vi "主界面.vi"() -> ()   [LabVIEW 2010]
uses:
  全局量/试验配置信息.vi
  全局量/全局_配置.vi
  全局量/自动测试结果.vi
panel:
  out "配置文件路径 2":path
  out "配置文件目录 2":path
  in  "进度提示":string
  in  "加载配置文件列表":u16(ring)
  out "配置文件路径":path
  out "配置文件目录":path
  in  "通道及参数配置":bool
  in  "选项卡":enum32{"板卡类型I", "板卡类型II"}(tab)
  in  "单选_数字量输入":bool
  in  "单选_数字量输出":bool
  in  "单选_DSP输入":bool
  in  "单选_CAN检测":bool
  in  "单选_LAN检测":bool
  in  "单选_R232检测":bool
  in  "btn_数字输出":bool
  in  "btn_DSP输入":bool
  in  "btn_CAN总线":bool
  in  "btn_LAN总线":bool
  in  "btn_R232_485总线":bool
  in  "btn_开始检测":bool
  in  "btn_数字输入":bool
  in  "单选_R485检测":bool
  in  "单选_AD输入":bool
  out "数字量输入检测":bool
  out "数字量输出检测":bool
  out "模拟量DSP输入检测":bool
  out "模拟量AD输入检测":bool
  out "CAN总线检测":bool
  out "LAN总线检测":bool
  out "RS232总线检测":bool
  out "RS485总线检测":bool
  in  "btn_自动开始检测类型2":bool
  in  "函数类型 4":bool caption="y =f4(A1sin(2*π*A2)x+A3)"
  in  "函数类型 3":bool caption="y =f3(x)"
  in  "函数类型 2":bool caption="y =f2(x,A1,A2,t)"
  in  "函数类型 1":bool caption="y =f1(A1*x+A2)"
  out "函数类型4检测":bool
  out "函数类型3检测":bool
  out "函数类型2检测":bool
  out "函数类型1检测":bool
  in  "单选_函数类型4":bool
  in  "单选_函数类型3":bool
  in  "单选_函数类型2":bool
  in  "单选_函数类型1":bool
  in  "进度每次增加数":dbl
  in  "btn_二维码识别":bool
  out "退出？":bool
  in  "btn_退出":bool
  in  "btn_报告管理":bool
  in  "str_测试地点":string
  in  "str_测试人员":string
  in  "str_测试编号":string
  in  "str_报告编号":string
  # "板卡综合测试装置"
  # "板 卡 测 试 信 息"
  # "试验报告编号："
  # "测试板卡编号："
  # "板卡类型："
  # "测试人员："
  # "测试地点："
  # "自动测试"
  # "分步测试"
  # "测试\n项\n目"
  # "分步测试"
  # "自动测试"
  # "测试\n项\n目"
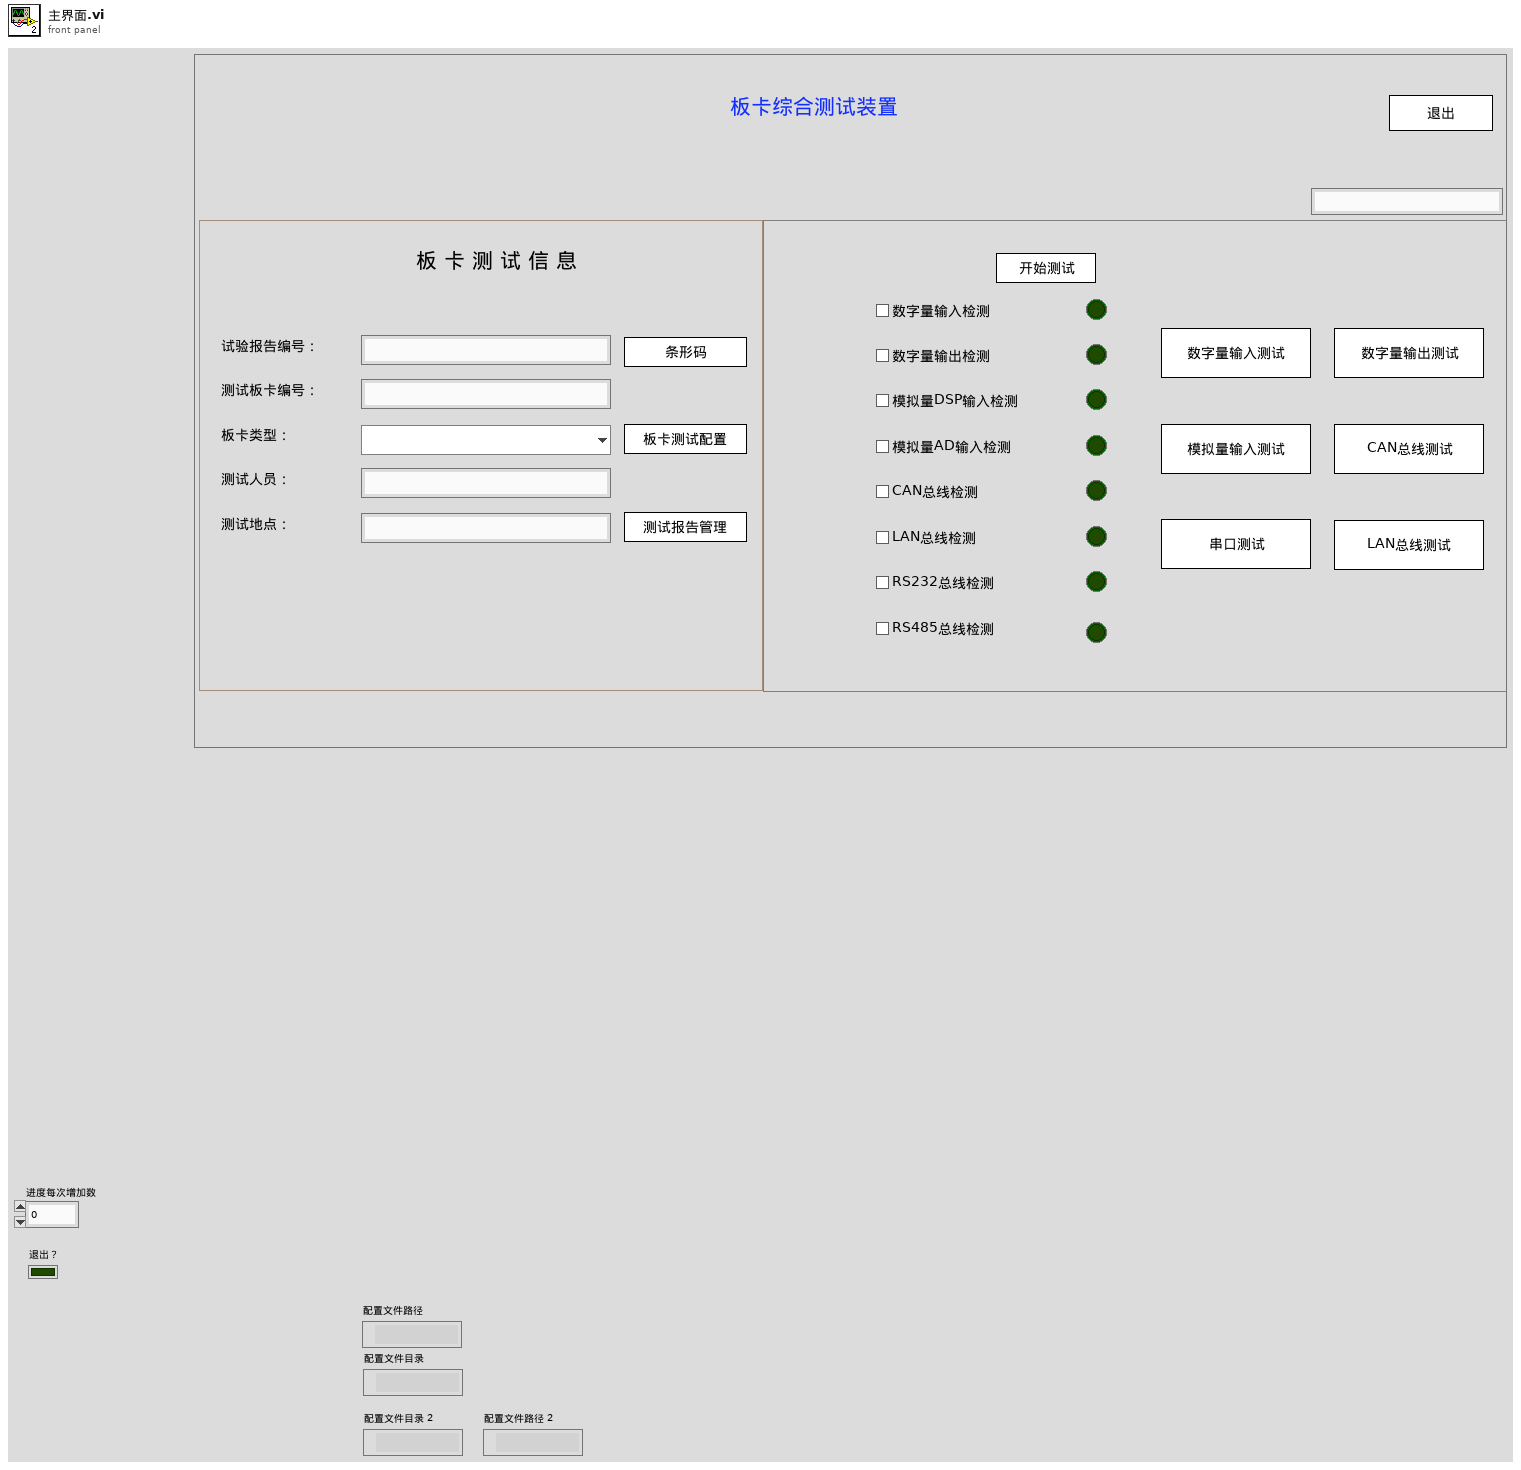
[diagram p1: front panel]
types:
  T1 = cluster{"数字量输入信号路数":i32, "数字量输出信号路数":i32, "DSP模拟量输入信号路数":u32, "DSP模拟量输入信号幅值":u32, "AD模拟量输入信号路数":u32, "AD模拟量输入信号幅值":u32, "RS232端口":u32, "RS232通信路数":u32, "RS232波特率":dbl, "RS485端口":u32, "RS485通信路数":u32, "RS485波特率":u32, "CAN通信路数":i32, "CAN波特率":u32, "以太网选择?":bool, "控制板IP":string, "以太网端口":u32}
  T2 = cluster{"str_报告编号":string, "str_测试编号":string, "RingText.Text":string, "str_测试人员":string, "str_测试地点":string}
  T3 = enum8{"Enabled", "Disabled", "Disabled and Grayed Out"}
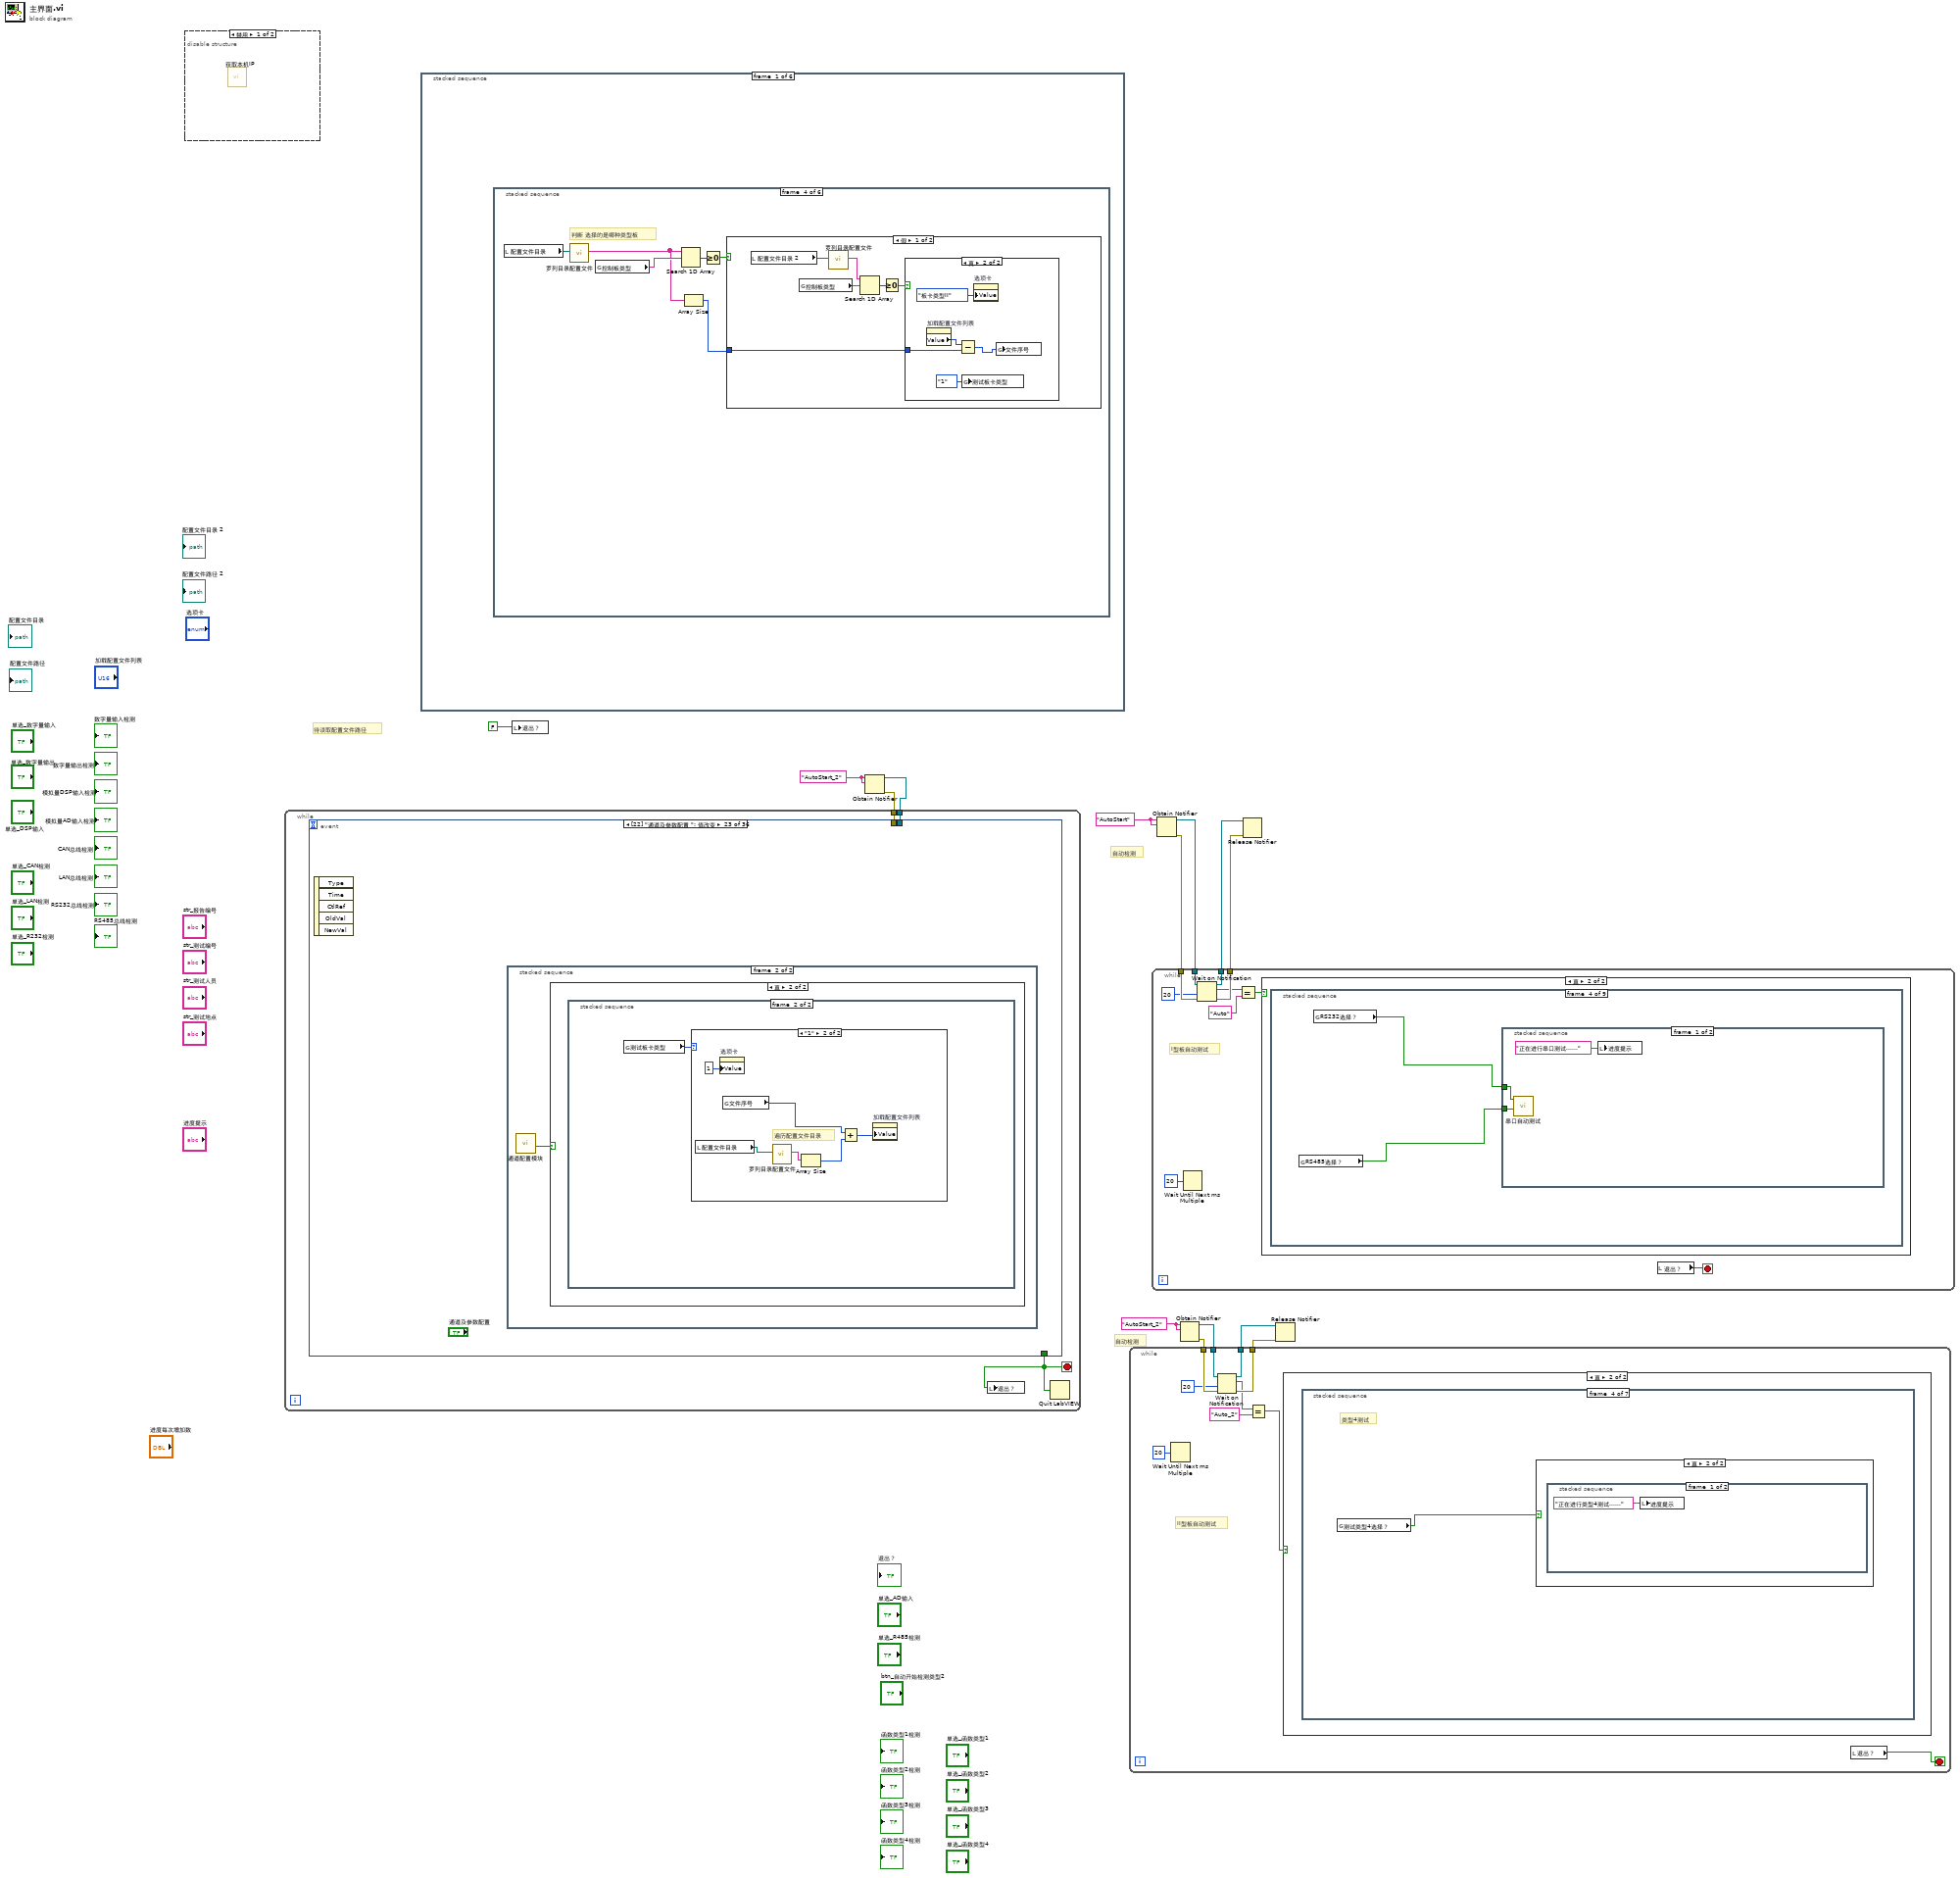
[diagram p0: block diagram]
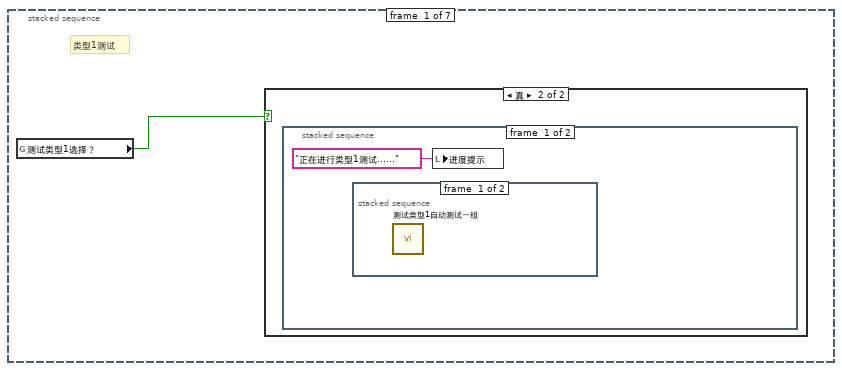
[diagram p4: hidden frame]
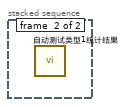
[diagram p6: hidden frame]
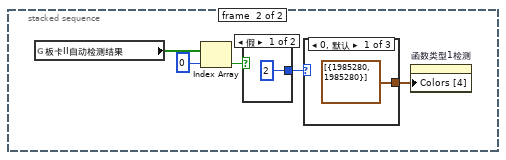
[diagram p7: hidden frame]
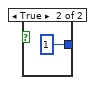
[diagram p8: hidden frame]
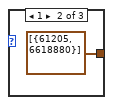
[diagram p9: hidden frame]
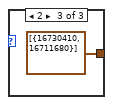
[diagram p10: hidden frame]
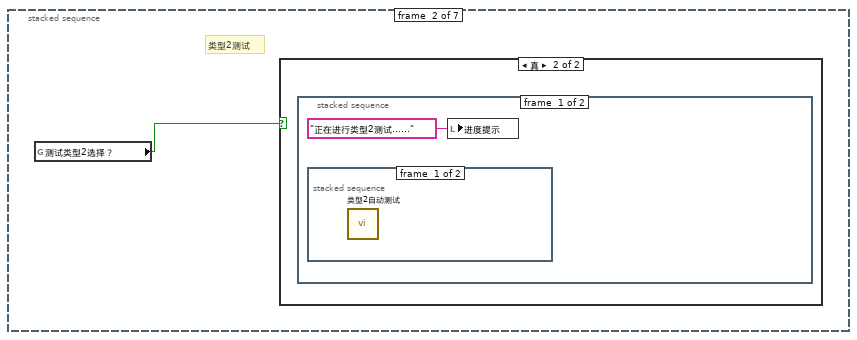
[diagram p11: hidden frame]
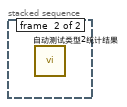
[diagram p13: hidden frame]
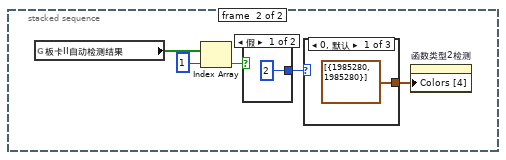
[diagram p14: hidden frame]
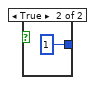
[diagram p15: hidden frame]
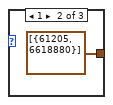
[diagram p16: hidden frame]
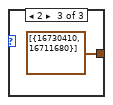
[diagram p17: hidden frame]
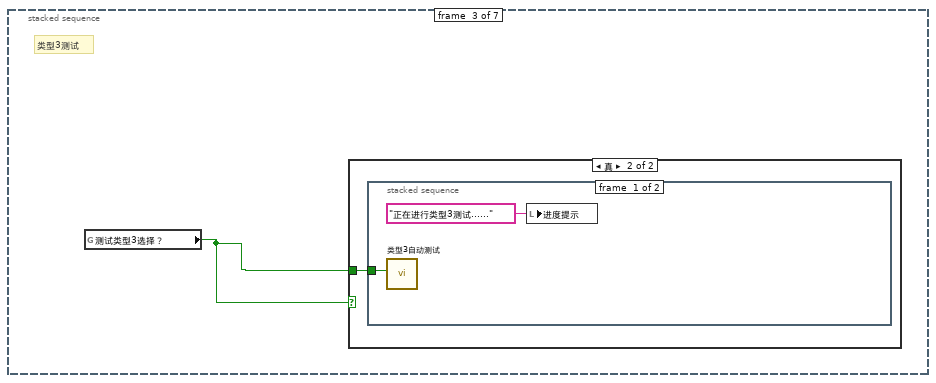
[diagram p18: hidden frame]
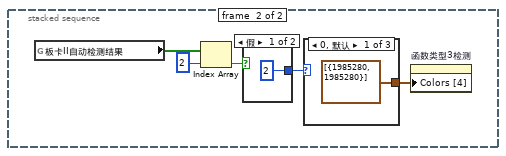
[diagram p20: hidden frame]
diagram:
  w4 = "AutoStart_2" ("名称（未命名）")
  w9 = "AutoStart_2" ("名称（未命名）")
  w14 = "AutoStart" ("名称（未命名）")
  # "待读取配置文件路径"
  # "自动检测"
  # "自动检测"
  n1 = disable-structure shown="禁用" {
    frame Disabled {
      n2 = call "获取本机IP.vi"() -> ()  [unwired: 9 in, 3 out]
    }
    frame Enabled {
    }
  }
  n3 = stacked-sequence {
    frame #0 {
      n4 = stacked-sequence {
        frame #0 {
          # "初始化配置文件路径"
          n5 = VI Library "VI库"() -> (path=w28:path)
          n6 = Strip Path(path=w28) -> (stripped path=w27:path)  [unwired: 1 out]
          n7 = Build Path(base path=w27, name or relative path="config" ("名称或相对路径")) -> (appended path=w16:path)
          n8 = Build Path(base path=w16, name or relative path="bordI_config" ("名称或相对路径")) -> (appended path=w22:path)
          n9 = Build Path(base path=w16, name or relative path="bordII_config" ("名称或相对路径")) -> (appended path=w19:path)
          n10 = call <vilib>:"Check if File or Folder Exists.vi"("path"=w22) -> ("file or folder exists?"=w23:bool, "dup path"=w24:path)  [unwired: 8 in, 1 out]
          n11 = call <vilib>:"Check if File or Folder Exists.vi"("path"=w19) -> ("file or folder exists?"=w18:bool, "dup path"=w17:path)  [unwired: 8 in, 1 out]
          n12 = case shown="假" w23 {
            tunnel: w24 -> [w32 w34]
            tunnel: [w33 w34] -> w21
            frame False {
              n13 = Create Folder(path (use dialog)=w32) -> (created path=w33:path)  [unwired: 2 in, 2 out]
            }
            frame True {
            }
          }
          n14 = case shown="假" w18 {
            tunnel: w17 -> [w29 w31]
            tunnel: [w30 w31] -> w20
            frame False {
              n15 = Create Folder(path (use dialog)=w29) -> (created path=w30:path)  [unwired: 2 in, 2 out]
            }
            frame True {
            }
          }
          n16 = local write "配置文件目录"(w21) -> ()
          n17 = local write "配置文件目录 2"(w20) -> ()
        }
        frame #1 {
          # "遍历配置文件目录"
          n18 = local read "配置文件目录"() -> (w39:path)
          n19 = local read "配置文件目录 2"() -> (w38:path)
          n20 = call "罗列目录配置文件.vi"("路径"=w39) -> ("数组"=w37:string[])  [unwired: 10 in]
          n21 = call "罗列目录配置文件.vi"("路径"=w38) -> ("数组"=w36:string[])  [unwired: 10 in]
          n22 = Insert Into Array(array=w37, new element=w36) -> (w35:string[])  [unwired: 1 in]
          n23 = property on="加载配置文件列表" class="Ring (严格)"("Strings []"=w35) -> ()  [unwired: 2 in, 2 out]
        }
        frame #2 {
          n24 = property on="加载配置文件列表" class="Ring (严格)"() -> ("RingText.Text"=w40:string)  [unwired: 2 in, 2 out]
          n25 = global write "试验配置信息.vi" "控制板类型"(w40) -> ()
        }
        frame #3 {
          # "判断 选择的是哪种类型板"
          n26 = local read "配置文件目录"() -> (w46:path)
          n27 = call "罗列目录配置文件.vi"("路径"=w46) -> ("数组"=w42:string[])  [unwired: 10 in]
          n28 = global read "试验配置信息.vi" "控制板类型"() -> (w45:string)
          n29 = Search 1D Array(1D array=w42, element=w45) -> (index of element=w44:i32)  [unwired: 1 in]
          n30 = Array Size(array=w42) -> (size(s)=w41:i32)
          n31 = Greater Or Equal To 0?(x=w44) -> (x >= 0?=w43:bool)
          n32 = case shown="假" w43 {
            tunnel: w41 -> [w47 _]
            frame False {
              n33 = local read "配置文件目录 2"() -> (w52:path)
              n34 = global read "试验配置信息.vi" "控制板类型"() -> (w51:string)
              n35 = call "罗列目录配置文件.vi"("路径"=w52) -> ("数组"=w50:string[])  [unwired: 10 in]
              n36 = Search 1D Array(1D array=w50, element=w51) -> (index of element=w49:i32)  [unwired: 1 in]
              n37 = Greater Or Equal To 0?(x=w49) -> (x >= 0?=w48:bool)
              n38 = case shown="真" w48 {
                tunnel: w47 -> [_ w54]
                frame False {
                }
                frame True {
                  n39 = property on="加载配置文件列表" class="Ring (严格)"() -> ("Value"=w56:u16)  [unwired: 2 in, 2 out]
                  n40 = Subtract(x=w56, y=w54) -> (x-y=w55:i32)
                  n41 = global write "试验配置信息.vi" "测试板卡类型"(enum16{"0", "1"}."1" ("测试板卡类型")) -> ()
                  n42 = property on="选项卡" class="TabCtl (严格)"("Value"=enum32{"板卡类型I", "板卡类型II"}."板卡类型II" ("选项卡")) -> ()  [unwired: 2 in, 2 out]
                  n43 = global write "试验配置信息.vi" "文件序号"(w55) -> ()
                }
              }
            }
            frame True {
              n44 = global write "试验配置信息.vi" "测试板卡类型"(enum16{"0", "1"}."0" ("测试板卡类型")) -> ()
              n45 = property on="选项卡" class="TabCtl (严格)"("Value"=enum32{"板卡类型I", "板卡类型II"}."板卡类型I" ("选项卡")) -> ()  [unwired: 2 in, 2 out]
              n46 = property on="加载配置文件列表" class="Ring (严格)"() -> ("Value"=w59:u16)  [unwired: 2 in, 2 out]
              n47 = global write "试验配置信息.vi" "文件序号"(w59) -> ()
            }
          }
        }
        frame #4 {
          # "待读取配置文件路径"
          n48 = local read "配置文件目录 2"() -> (w63:path)
          n49 = global read "试验配置信息.vi" "控制板类型"() -> (w61:string)
          n50 = Build Path(base path=w63, name or relative path=w61) -> (appended path=w62:path)
          n51 = local write "配置文件路径 2"(w62) -> ()
        }
        frame #5 {
          n52 = local read "配置文件路径 2"() -> (w66:path)
          n53 = call <vilib>:"Check if File or Folder Exists.vi"("path"=w66) -> ("file or folder exists?"=w65:bool, "dup path"=w64:path)  [unwired: 8 in, 1 out]
          n54 = case shown="真" w65 {
            tunnel: w64 -> [_ w67]
            frame False {
            }
            frame True {
              n55 = call "函数测试配置文件读取.vi"("配置文件路径"=w67) -> ("类型1路数"=w71:i32, "类型2路数"=w70:i32, "类型3路数"=w69:i32, "类型4路数"=w68:i32, "D_IN_1"=w75:string[][], "D_IN_2"=w74:string[][], "D_IN_3"=w73:string[][], "D_IN_4"=w72:string[][])  [unwired: 11 in]
              n56 = global write "试验配置信息.vi" "自测类型4路数"(w68) -> ()
              n57 = global write "试验配置信息.vi" "D_IN_1"(w75) -> ()
              n58 = global write "试验配置信息.vi" "D_IN_2"(w74) -> ()
              n59 = global write "试验配置信息.vi" "D_IN_3"(w73) -> ()
              n60 = global write "试验配置信息.vi" "D_IN_4"(w72) -> ()
              n61 = global write "试验配置信息.vi" "自测类型1路数"(w71) -> ()
              n62 = global write "试验配置信息.vi" "自测类型2路数"(w70) -> ()
              n63 = global write "试验配置信息.vi" "自测类型3路数"(w69) -> ()
            }
          }
        }
      }
    }
    frame #1 {
      n64 = global read "试验配置信息.vi" "控制板类型"() -> (w78:string)
      n65 = global write "全局_配置.vi" "CAN打开标志"(FALSE ("CAN打开标志")) -> ()
      n66 = local write "加载配置文件列表"(u16 0) -> ()
      n67 = call "读写配置文件.vi"("m_bCreat"=FALSE, "文件名称"=w78, "m_bRead"=TRUE) -> ("BoardConfig_output"=w92:T1)  [unwired: 8 in]
      n68 = Unbundle By Name(w92) -> ("数字量输入信号路数"=w86:i32, "数字量输出信号路数"=w85:i32, "DSP模拟量输入信号路数"=w84:u32, "DSP模拟量输入信号幅值"=w90:u32, "AD模拟量输入信号路数"=w83:u32, "AD模拟量输入信号幅值"=w87:u32, "RS232通信路数"=w82:u32, "RS232波特率"=w91:dbl, "RS485通信路数"=w81:u32, "CAN通信路数"=w80:i32)  [unwired: 7 out]
      n69 = global write "全局_配置.vi" "BoardConfig"(w92) -> ()
      n70 = global write "试验配置信息.vi" "测试板卡类型"(enum16{"0", "1"}."0" ("测试板卡类型")) -> ()
      n71 = case shown="0, 默认" w90 {
        tunnel: [3.3 10.0 24.0] -> w89
        frame 0, Default {
        }
        frame 1 {
        }
        frame 2 {
        }
      }
      n72 = case shown="2" w87 {
        tunnel: [6.0 10.0 24.0] -> w88
        frame 0, Default {
        }
        frame 1 {
        }
        frame 2 {
        }
      }
      n73 = global write "全局_配置.vi" "模拟量误差"(w91) -> ()
      n74 = global write "全局_配置.vi" "数字量输入路数"(w86) -> ()
      n75 = global write "全局_配置.vi" "数字量输出路数"(w85) -> ()
      n76 = global write "全局_配置.vi" "dsp模拟量输入路数"(w84) -> ()
      n77 = global write "全局_配置.vi" "ad模拟量输入路数"(w83) -> ()
      n78 = global write "试验配置信息.vi" "自测CAN路数"(w80) -> ()
      n79 = global write "全局_配置.vi" "R485路数"(w81) -> ()
      n80 = global write "全局_配置.vi" "CAN波特率"(u16 250 ("CAN波特率")) -> ()
      n81 = global write "全局_配置.vi" "R232路数"(w82) -> ()
      n82 = global write "全局_配置.vi" "DSP模拟量量程范围"(w89) -> ()
      n83 = global write "全局_配置.vi" "ARM模拟量量程范围"(w88) -> ()
      n84 = disable-structure shown="禁用" {
        frame Disabled {
          (unwired) "192.168.1.15" ("本机IP")
          (unwired) "192.168.1.10" ("控制板IP")
        }
        frame Enabled {
        }
      }
      n85 = global write "全局_配置.vi" "CAN发送帧数"(u32 100 ("CAN发送帧数")) -> ()
      n86 = global write "全局_配置.vi" "超时时间_10"(2.0 ("超时时间_102")) -> ()
      n87 = global write "全局_配置.vi" "超时时间_2"(2.0 ("超时时间_2")) -> ()
      n88 = global write "全局_配置.vi" "控制板端口"(u16 6600 ("控制板端口")) -> ()
      n89 = global write "全局_配置.vi" "本机端口"(u16 6601 ("本机端口")) -> ()
      n90 = global write "全局_配置.vi" "本机IP"("192.168.1.15" ("本机IP")) -> ()
      n91 = global write "全局_配置.vi" "控制板IP"("192.168.1.10" ("控制板IP")) -> ()
    }
    frame #2 {
      n92 = global write "试验配置信息.vi" "自测485路数"(1 ("自测485路数")) -> ()
      n93 = global write "试验配置信息.vi" "自测LAN路数"(1 ("自测LAN路数")) -> ()
    }
    frame #3 {
      w140 = TRUE ("单选_数字量输入")
      # "自动测试"
      n94 = case shown="0, 默认" 0 {
        tunnel: [cluster{u32, u32}[] [{1985280, 1985280}] cluster{u32, u32}[] [{61205, 6618880}] cluster{u32, u32}[] [{16730410, 16711680}]] -> w139
        frame 0, Default {
        }
        frame 1 {
        }
        frame 2 {
        }
      }
      n95 = property on="数字量输入检测" class="Bool (严格)"("Colors [4]"=w139) -> ()  [unwired: 2 in, 2 out]
      n96 = property on="数字量输出检测" class="Bool (严格)"("Colors [4]"=w139) -> ()  [unwired: 2 in, 2 out]
      n97 = property on="模拟量AD输入检测" class="Bool (严格)"("Colors [4]"=w139) -> ()  [unwired: 2 in, 2 out]
      n98 = property on="CAN总线检测" class="Bool (严格)"("Colors [4]"=w139) -> ()  [unwired: 2 in, 2 out]
      n99 = global write "自动测试结果.vi" "DI自动测试结果"(string[][] [["序号", "检测内容", "结果"]] ("自动测试结果")) -> ()
      n100 = property on="LAN总线检测" class="Bool (严格)"("Colors [4]"=w139) -> ()  [unwired: 2 in, 2 out]
      n101 = property on="RS232总线检测" class="Bool (严格)"("Colors [4]"=w139) -> ()  [unwired: 2 in, 2 out]
      n102 = property on="RS485总线检测" class="Bool (严格)"("Colors [4]"=w139) -> ()  [unwired: 2 in, 2 out]
      n103 = property on="模拟量DSP输入检测" class="Bool (严格)"("Colors [4]"=w139) -> ()  [unwired: 2 in, 2 out]
      n104 = property on="函数类型1检测" class="Bool (严格)"("Colors [4]"=w139) -> ()  [unwired: 2 in, 2 out]
      n105 = property on="函数类型2检测" class="Bool (严格)"("Colors [4]"=w139) -> ()  [unwired: 2 in, 2 out]
      n106 = property on="函数类型3检测" class="Bool (严格)"("Colors [4]"=w139) -> ()  [unwired: 2 in, 2 out]
      n107 = property on="函数类型4检测" class="Bool (严格)"("Colors [4]"=w139) -> ()  [unwired: 2 in, 2 out]
      n108 = global write "试验配置信息.vi" "自测类数"(0 ("自动测试个数")) -> ()
      n109 = local write "str_报告编号"("B001001000001" ("通知")) -> ()
      n110 = local write "str_测试地点"("1号实验室" ("str_测试地点")) -> ()
      n111 = global read "试验配置信息.vi" "自测类型1路数"() -> (w126:i32)
      n112 = global read "试验配置信息.vi" "自测类型1路数"() -> (w137:i32)
      n113 = global read "试验配置信息.vi" "自测类型2路数"() -> (w134:i32)
      n114 = global read "试验配置信息.vi" "自测类型3路数"() -> (w131:i32)
      n115 = global read "试验配置信息.vi" "自测类型4路数"() -> (w128:i32)
      n116 = Initialize Array(TRUE, 5 ("维数大小"), 16 ("维数大小")) -> (w116:bool[][])
      n117 = Initialize Array(TRUE, 5 ("维数大小"), 16 ("维数大小")) -> (w121:bool[][])
      n118 = Initialize Array(0.0, w126) -> (w125:dbl[])
      n119 = Initialize Array(TRUE ("元素"), w137) -> (w138:bool[])
      n120 = Initialize Array(TRUE ("元素"), w134) -> (w133:bool[])
      n121 = Initialize Array(TRUE ("元素"), w131) -> (w132:bool[])
      n122 = Initialize Array(TRUE ("元素"), w128) -> (w127:bool[])
      n123 = Initialize Array(TRUE ("元素"), 4 ("维数大小")) -> (w146:bool[])
      n124 = Initialize Array(TRUE ("元素"), 1 ("维数大小")) -> (w145:bool[])
      n125 = local write "单选_数字量输入"(w140) -> ()
      n126 = local write "单选_数字量输出"(w140) -> ()
      n127 = local write "单选_DSP输入"(w140) -> ()
      n128 = local write "单选_CAN检测"(w140) -> ()
      n129 = local write "单选_LAN检测"(w140) -> ()
      n130 = local write "单选_R232检测"(w140) -> ()
      n131 = local write "单选_R485检测"(w140) -> ()
      n132 = local write "单选_AD输入"(w140) -> ()
      n133 = Initialize Array(TRUE ("元素"), 16 ("维数大小")) -> (w153:bool[])
      n134 = Initialize Array(TRUE ("元素"), 2 ("维数大小")) -> (w142:bool[])
      n135 = Initialize Array(TRUE ("元素"), 16 ("维数大小")) -> (w148:bool[])
      n136 = global write "自动测试结果.vi" "Auto_DO_R"(w116) -> ()
      n137 = global write "自动测试结果.vi" "Auto_DI_R"(w121) -> ()
      n138 = global write "自动测试结果.vi" "Auto_func_1_max_WC"(w125) -> ()
      n139 = global write "自动测试结果.vi" "Auto_func_1_R"(w138) -> ()
      n140 = global write "自动测试结果.vi" "Auto_func_2_R"(w133) -> ()
      n141 = global write "自动测试结果.vi" "Auto_func_3_R"(w132) -> ()
      n142 = global write "自动测试结果.vi" "Auto_func_4_R"(w127) -> ()
      n143 = global write "自动测试结果.vi" "Auto_RS485_R"(w145) -> ()
      n144 = global write "自动测试结果.vi" "Auto_RS232_R"(w142) -> ()
      n145 = global write "自动测试结果.vi" "Auto_CAN_R"(w146) -> ()
      n146 = global write "自动测试结果.vi" "Auto_DSP_R"(w153) -> ()
      n147 = global write "自动测试结果.vi" "Auto_AD_R"(w148) -> ()
      n148 = local write "单选_函数类型1"(w140) -> ()
      n149 = local write "单选_函数类型2"(w140) -> ()
      n150 = local write "单选_函数类型3"(w140) -> ()
      n151 = local write "单选_函数类型4"(w140) -> ()
    }
    frame #4 {
      n152 = call "实验配置信息读取和写入.vi"("读取写入"=FALSE) -> ("输出簇"=w175:T2)  [unwired: 8 in]
      n153 = Unbundle By Name(w175) -> ("str_报告编号"=w173:string, "str_测试编号"=w172:string, "str_测试人员"=w170:string, "str_测试地点"=w171:string)
      n154 = Initialize Array(TRUE, 8 ("维数大小")) -> (w168:bool[])
      n155 = Initialize Array(TRUE, 4 ("维数大小")) -> (w165:bool[])
      n156 = call <vilib>:"RGB to Color.vi"("B"=255 ("维数大小"), "G"=0 ("维数大小"), "R"=0 ("维数大小")) -> ("Color"=w162:u32)
      n157 = global write "试验配置信息.vi" "板卡II自动检测结果"(w165) -> ()
      n158 = local write "str_报告编号"(w173) -> ()
      n159 = local write "str_测试编号"(w172) -> ()
      n160 = property on="进度提示" class="Str"("Text.TextColor"=w162) -> ()  [unwired: 2 in, 2 out]
      n161 = local write "进度提示"("测试准备就绪......") -> ()
      n162 = global write "试验配置信息.vi" "自动检测结果"(w168) -> ()
      n163 = local write "str_测试地点"(w171) -> ()
      n164 = local write "str_测试人员"(w170) -> ()
    }
    frame #5 {
      n165 = local read "str_测试编号"() -> (w176:string)
      n166 = global write "试验配置信息.vi" "条形码"(w176) -> ()
    }
  }
  n167 = local write "退出？"(FALSE) -> ()
  n168 = Obtain Notifier(name (unnamed)=w4, notification data type=w4) -> (notifier out=w3:refnum<notifier>, error out=w2:errorcluster)  [unwired: 2 in, 1 out]
  n169 = while {
    tunnel: w3 -> [w178]
    tunnel: w2 -> [w177]
    stop <- w179 stop-if-true
    n170 = event shown="[22] \"通道及参数配置 \": 值改变" {
      selector: _ -> [_ _ _ _ _ _ _ _ _ _ _ _ _ _ _ _ _ _ _ _ _ _ _ _ _ _ _ _ _ _ _ _ _ _ _ _]
      dyn-events: _ -> [_ _ _ _ _ _ _ _ _ _ _ _ _ _ _ _ _ _ _ _ _ _ _ _ _ _ _ _ _ _ _ _ _ _ _ _]
      timeout: _ -> [_ _ _ _ _ _ _ _ _ _ _ _ _ _ _ _ _ _ _ _ _ _ _ _ _ _ _ _ _ _ _ _ _ _ _ _]
      tunnel: [_ w180 _ _ _ _ _ _ _ _ _ _ _ _ _ _ _ _ _ _ _ _ _ _ _ _ _ _ _ _ _ _ _ _ _ _] -> w179
      tunnel: w178 -> [_ _ _ _ _ _ _ _ _ _ _ _ _ _ _ _ _ w407 _ _ _ _ _ _ _ _ _ _ _ _ _ _ _ _ _ _]
      tunnel: w177 -> [_ _ _ _ _ _ _ _ _ _ _ _ _ _ _ _ _ w406 _ _ _ _ _ _ _ _ _ _ _ _ _ _ _ _ _ _]
      event Timeout {
        n171 = event-data() -> ()  [unwired: 1 in, 2 out]
      }
      event "btn_退出": Value Change {
        n172 = event-data() -> ()  [unwired: 1 in, 5 out]
        n173 = case shown="真" "btn_退出" {
          tunnel: [FALSE TRUE] -> w180
          frame False {
          }
          frame True {
          }
        }
      }
      event "btn_报告管理": Value Change {
        n174 = event-data() -> ()  [unwired: 1 in, 5 out]
        n175 = call "测试报告管理.vi"() -> ()  [unwired: 12 in]
      }
      event "单选_数字量输入": Value Change {
        n176 = event-data() -> ("NewVal"=w184:bool)  [unwired: 1 in, 4 out]
        n177 = local write "单选_数字量输入"(w184) -> ()
      }
      event "单选_数字量输出": Value Change {
        n178 = event-data() -> ("NewVal"=w185:bool)  [unwired: 1 in, 4 out]
        n179 = local write "单选_数字量输出"(w185) -> ()
      }
      event "单选_DSP输入": Value Change {
        n180 = event-data() -> ("NewVal"=w186:bool)  [unwired: 1 in, 4 out]
        n181 = local write "单选_DSP输入"(w186) -> ()
      }
      event "单选_CAN检测": Value Change {
        n182 = event-data() -> ("NewVal"=w187:bool)  [unwired: 1 in, 4 out]
        n183 = local write "单选_CAN检测"(w187) -> ()
      }
      event "单选_LAN检测": Value Change {
        n184 = event-data() -> ("NewVal"=w188:bool)  [unwired: 1 in, 4 out]
        n185 = local write "单选_LAN检测"(w188) -> ()
      }
      event "单选_R232检测": Value Change {
        n186 = event-data() -> ("NewVal"=w189:bool)  [unwired: 1 in, 4 out]
        n187 = local write "单选_R232检测"(w189) -> ()
      }
      event "btn_数字输入": Value Change {
        n188 = event-data() -> ()  [unwired: 1 in, 5 out]
        n189 = call "数字量输入配置.vi"() -> ()  [unwired: 12 in]
      }
      event "btn_数字输出": Value Change {
        n190 = event-data() -> ()  [unwired: 1 in, 5 out]
        n191 = call "数字量输出配置.vi"() -> ()  [unwired: 12 in]
      }
      event "btn_DSP输入": Value Change {
        n192 = event-data() -> ()  [unwired: 1 in, 5 out]
        n193 = call "32路模拟量输入.vi"() -> ()  [unwired: 12 in]
      }
      event "btn_CAN总线": Value Change {
        n194 = event-data() -> ()  [unwired: 1 in, 5 out]
        n195 = call "CAN总线测试.vi"() -> ()  [unwired: 12 in]
      }
      event "btn_LAN总线": Value Change {
        n196 = event-data() -> ()  [unwired: 1 in, 5 out]
        n197 = call "以太网测试界面.vi"() -> ()  [unwired: 12 in]
      }
      event "btn_R232_485总线": Value Change {
        n198 = event-data() -> ()  [unwired: 1 in, 5 out]
        n199 = call "RS232 485发送接收.vi"() -> ()  [unwired: 12 in]
      }
      event "btn_开始检测": Value Change {
        w191 = ""
        n200 = event-data() -> ()  [unwired: 1 in, 5 out]
        n201 = local read "单选_数字量输入"() -> (w200:bool)
        n202 = local read "单选_数字量输出"() -> (w199:bool)
        n203 = local read "单选_R232检测"() -> (w195:bool)
        n204 = local read "单选_R485检测"() -> (w196:bool)
        n205 = local read "单选_CAN检测"() -> (w193:bool)
        n206 = local read "单选_LAN检测"() -> (w194:bool)
        n207 = local read "单选_DSP输入"() -> (w198:bool)
        n208 = local read "单选_AD输入"() -> (w197:bool)
        n209 = local read "str_报告编号"() -> (w211:string)
        n210 = local read "str_测试编号"() -> (w210:string)
        n211 = local read "str_测试地点"() -> (w209:string)
        n212 = local read "str_测试人员"() -> (w208:string)
        n213 = property on="加载配置文件列表" class="Ring (严格)"() -> ("RingText.Text"=w192:string)  [unwired: 2 in, 2 out]
        n214 = Not Equal?(x=w211, y=w191) -> (x != y?=w207:bool)
        n215 = Not Equal?(x=w210, y=w191) -> (x != y?=w206:bool)
        n216 = Not Equal?(x=w209, y=w191) -> (x != y?=w205:bool)
        n217 = Not Equal?(x=w208, y=w191) -> (x != y?=w204:bool)
        n218 = Not Equal?(x=w192, y=w191) -> (x != y?=w190:bool)
        n219 = global write "试验配置信息.vi" "数字量输出选择？"(w199) -> ()
        n220 = global write "试验配置信息.vi" "数字量输入选择？"(w200) -> ()
        n221 = Compound Arithmetic op=AND(w190, w207, w206, w205, w204) -> (w202:bool)
        n222 = global write "试验配置信息.vi" "DSP输入选择？"(w198) -> ()
        n223 = global write "试验配置信息.vi" "CAN选择？"(w193) -> ()
        n224 = global write "试验配置信息.vi" "LAN选择？"(w194) -> ()
        n225 = global write "试验配置信息.vi" "RS232选择？"(w195) -> ()
        n226 = global write "试验配置信息.vi" "RS485选择？"(w196) -> ()
        n227 = global write "试验配置信息.vi" "AD输入选择？"(w197) -> ()
        n228 = Compound Arithmetic op=OR(w200, w199, w198, w193, w194, w195, w196, w197) -> (w201:bool)
        n229 = And(x=w202, y=w201) -> (x .and. y?=w203:bool)
        n230 = case shown="真" w203 {
          tunnel: w202 -> [w213 _]
          tunnel: w201 -> [w212 _]
          frame False {
            n231 = case shown="假" w212 {
              frame False {
                n232 = call "显示对话框信息2"() -> ()  [unwired: 10 in, 2 out]
              }
              frame True {
              }
            }
            n233 = case shown="假" w213 {
              frame False {
                n234 = call "显示对话框信息"() -> ()  [unwired: 10 in, 2 out]
              }
              frame True {
              }
            }
          }
          frame True {
            n235 = stacked-sequence {
              frame #0 {
                n236 = property on="加载配置文件列表" class="Ring (严格)"() -> ("RingText.Text"=w217:string)  [unwired: 2 in, 2 out]
                n237 = local read "str_报告编号"() -> (w223:string)
                n238 = local read "str_测试编号"() -> (w224:string)
                n239 = local read "str_测试地点"() -> (w226:string)
                n240 = local read "str_测试人员"() -> (w225:string)
                n241 = local read "str_测试地点"() -> (w216:string)
                n242 = local read "str_报告编号"() -> (w221:string)
                n243 = local read "str_测试编号"() -> (w220:string)
                n244 = local read "str_测试人员"() -> (w218:string)
                n245 = global write "试验配置信息.vi" "自测类数"(0 ("自测类数")) -> ()
                n246 = global write "试验配置信息.vi" "自测项数"(0 ("自测类数")) -> ()
                n247 = global write "试验配置信息.vi" "报告编号"(w223) -> ()
                n248 = global write "试验配置信息.vi" "控制板编号"(w224) -> ()
                n249 = global write "试验配置信息.vi" "测试地点"(w226) -> ()
                n250 = global write "试验配置信息.vi" "测试人员"(w225) -> ()
                n251 = Bundle("str_报告编号"=w221, "str_测试编号"=w220, "RingText.Text"=w217, "str_测试人员"=w218, "str_测试地点"=w216) -> (w219:T2)  [unwired: 1 in]
                n252 = global write "试验配置信息.vi" "控制板类型"(w217) -> ()
                n253 = call "实验配置信息读取和写入.vi"("读取写入"=TRUE, "输入簇"=w219) -> ()  [unwired: 7 in, 1 out]
              }
              frame #1 {
                n254 = stacked-sequence {
                  frame #0 {
                    n255 = local read "单选_数字量输入"() -> (w228:bool)
                    n256 = global read "全局_配置.vi" "数字量输入路数"() -> (w230:i32)
                    n257 = Greater Than 0?(x=w230) -> (x > 0?=w229:bool)
                    n258 = And(x=w229, y=w228) -> (x .and. y?=w227:bool)
                    n259 = global write "试验配置信息.vi" "数字量输入选择？"(w227) -> ()
                  }
                  frame #1 {
                    n260 = local read "单选_数字量输出"() -> (w232:bool)
                    n261 = global read "全局_配置.vi" "数字量输出路数"() -> (w234:i32)
                    n262 = Greater Than 0?(x=w234) -> (x > 0?=w233:bool)
                    n263 = And(x=w233, y=w232) -> (x .and. y?=w231:bool)
                    n264 = global write "试验配置信息.vi" "数字量输出选择？"(w231) -> ()
                  }
                  frame #2 {
                    n265 = local read "单选_DSP输入"() -> (w236:bool)
                    n266 = global read "全局_配置.vi" "dsp模拟量输入路数"() -> (w238:u32)
                    n267 = Greater Than 0?(x=w238) -> (x > 0?=w237:bool)
                    n268 = And(x=w237, y=w236) -> (x .and. y?=w235:bool)
                    n269 = global write "试验配置信息.vi" "DSP输入选择？"(w235) -> ()
                  }
                  frame #3 {
                    n270 = local read "单选_AD输入"() -> (w240:bool)
                    n271 = global read "全局_配置.vi" "ad模拟量输入路数"() -> (w242:u32)
                    n272 = Greater Than 0?(x=w242) -> (x > 0?=w241:bool)
                    n273 = And(x=w241, y=w240) -> (x .and. y?=w239:bool)
                    n274 = global write "试验配置信息.vi" "AD输入选择？"(w239) -> ()
                  }
                  frame #4 {
                    n275 = global read "试验配置信息.vi" "自测CAN路数"() -> (w243:i32)
                    n276 = local read "单选_CAN检测"() -> (w245:bool)
                    n277 = Greater Than 0?(x=w243) -> (x > 0?=w246:bool)
                    n278 = And(x=w246, y=w245) -> (x .and. y?=w244:bool)
                    n279 = global write "试验配置信息.vi" "CAN选择？"(w244) -> ()
                  }
                  frame #5 {
                    n280 = global read "全局_配置.vi" "R232路数"() -> (w247:u32)
                    n281 = local read "单选_R232检测"() -> (w249:bool)
                    n282 = Greater Than 0?(x=w247) -> (x > 0?=w250:bool)
                    n283 = And(x=w250, y=w249) -> (x .and. y?=w248:bool)
                    n284 = global write "试验配置信息.vi" "RS232选择？"(w248) -> ()
                  }
                  frame #6 {
                    n285 = global read "全局_配置.vi" "R485路数"() -> (w251:u32)
                    n286 = local read "单选_R485检测"() -> (w253:bool)
                    n287 = Greater Than 0?(x=w251) -> (x > 0?=w254:bool)
                    n288 = And(x=w254, y=w253) -> (x .and. y?=w252:bool)
                    n289 = global write "试验配置信息.vi" "RS485选择？"(w252) -> ()
                  }
                }
              }
              frame #2 {
                n290 = global read "试验配置信息.vi" "数字量输入选择？"() -> (w262:bool)
                n291 = global read "试验配置信息.vi" "数字量输出选择？"() -> (w261:bool)
                n292 = global read "试验配置信息.vi" "DSP输入选择？"() -> (w260:bool)
                n293 = global read "试验配置信息.vi" "AD输入选择？"() -> (w255:bool)
                n294 = global read "试验配置信息.vi" "RS232选择？"() -> (w257:bool)
                n295 = global read "试验配置信息.vi" "RS485选择？"() -> (w256:bool)
                n296 = global read "试验配置信息.vi" "CAN选择？"() -> (w259:bool)
                n297 = global read "试验配置信息.vi" "LAN选择？"() -> (w258:bool)
                n298 = Build Array(w262, w261, w260, w259, w258, w257, w256, w255) -> (w263:bool[])
                n299 = for {
                  tunnel: w263 -> [w264] mode=indexing
                  n300 = case shown="真" w264 {
                    frame False {
                    }
                    frame True {
                      n301 = global read "试验配置信息.vi" "自测类数"() -> (w266:i32)
                      n302 = Increment(x=w266) -> (x+1=w265:i32)
                      n303 = global write "试验配置信息.vi" "自测类数"(w265) -> ()
                    }
                  }
                }
              }
              frame #3 {
                n304 = global read "试验配置信息.vi" "数字量输出选择？"() -> (w273:bool)
                n305 = global read "试验配置信息.vi" "数字量输入选择？"() -> (w274:bool)
                n306 = global read "试验配置信息.vi" "AD输入选择？"() -> (w271:bool)
                n307 = global read "试验配置信息.vi" "DSP输入选择？"() -> (w272:bool)
                n308 = global read "试验配置信息.vi" "CAN选择？"() -> (w270:bool)
                n309 = global read "试验配置信息.vi" "RS232选择？"() -> (w268:bool)
                n310 = global read "试验配置信息.vi" "RS485选择？"() -> (w267:bool)
                n311 = global read "试验配置信息.vi" "LAN选择？"() -> (w269:bool)
                n312 = case shown="真" w272 {
                  tunnel: [0 w293] -> w280
                  frame False {
                  }
                  frame True {
                    n313 = global read "全局_配置.vi" "dsp模拟量输入路数"() -> (w293:u32)
                  }
                }
                n314 = case shown="真" w271 {
                  tunnel: [0 w295] -> w281
                  frame False {
                  }
                  frame True {
                    n315 = global read "全局_配置.vi" "ad模拟量输入路数"() -> (w295:u32)
                  }
                }
                n316 = case shown="真" w273 {
                  tunnel: [0 w297] -> w282
                  frame False {
                  }
                  frame True {
                    n317 = global read "全局_配置.vi" "数字量输出路数"() -> (w297:i32)
                  }
                }
                n318 = case shown="真" w274 {
                  tunnel: [0 w299] -> w283
                  frame False {
                  }
                  frame True {
                    n319 = global read "全局_配置.vi" "数字量输入路数"() -> (w299:i32)
                  }
                }
                n320 = case shown="真" w270 {
                  tunnel: [0 w291] -> w279
                  frame False {
                  }
                  frame True {
                    n321 = global read "试验配置信息.vi" "自测CAN路数"() -> (w291:i32)
                  }
                }
                n322 = case shown="真" w268 {
                  tunnel: [0 w289] -> w278
                  frame False {
                  }
                  frame True {
                    n323 = global read "全局_配置.vi" "R232路数"() -> (w289:u32)
                  }
                }
                n324 = case shown="真" w267 {
                  tunnel: [0 w287] -> w277
                  frame False {
                  }
                  frame True {
                    n325 = global read "试验配置信息.vi" "自测485路数"() -> (w287:i32)
                  }
                }
                n326 = case shown="真" w269 {
                  tunnel: [0 w285] -> w276
                  frame False {
                  }
                  frame True {
                    n327 = global read "试验配置信息.vi" "自测LAN路数"() -> (w285:i32)
                  }
                }
                n328 = Compound Arithmetic op=ADD(w283, w282, w281, w280, w279, w278, w277, w276) -> (w275:u32)
                n329 = global write "试验配置信息.vi" "自测项数"(w275) -> ()
              }
              frame #4 {
                w307 = string[][] [["序号", "检测内容", "测试结果"]] ("自动测试结果")
                n330 = global read "全局_配置.vi" "dsp模拟量输入路数"() -> (w300:u32)
                n331 = global read "全局_配置.vi" "ad模拟量输入路数"() -> (w301:u32)
                n332 = Initialize Array(0.0 ("元素"), w300) -> (w302:dbl[])
                n333 = Initialize Array(0.0 ("元素"), w301) -> (w304:dbl[])
                n334 = global write "自动测试结果.vi" "总线通信自测结果"(w307) -> ()
                n335 = global write "自动测试结果.vi" "DI自动测试结果"(w307) -> ()
                n336 = global write "自动测试结果.vi" "DO自动测试结果"(w307) -> ()
                n337 = global write "自动测试结果.vi" "Auto_DSP_max_WC"(w302) -> ()
                n338 = global write "自动测试结果.vi" "Auto_AD_max_WC"(w304) -> ()
                n339 = global write "自动测试结果.vi" "AI自动测试结果"(string[][] [["序号", "检测内容", "最大误差(%)", "测试结果"]] ("自动测试结果")) -> ()
              }
              frame #5 {
                n340 = global read "试验配置信息.vi" "自测CAN路数"() -> (w324:i32)
                n341 = global read "试验配置信息.vi" "自测485路数"() -> (w327:i32)
                n342 = Initialize Array(TRUE ("元素"), w324) -> (w325:bool[])
                n343 = Initialize Array(TRUE ("元素"), w327) -> (w326:bool[])
                n344 = Initialize Array(TRUE ("元素"), 16 ("维数大小")) -> (w320:bool[])
                n345 = Initialize Array(TRUE ("元素"), 2 ("维数大小")) -> (w330:bool[])
                n346 = Initialize Array(TRUE ("元素"), 16 ("维数大小")) -> (w322:bool[])
                n347 = Initialize Array(TRUE, 5 ("维数大小"), 16 ("维数大小")) -> (w314:bool[][])
                n348 = Initialize Array(TRUE, 5 ("维数大小"), 16 ("维数大小")) -> (w318:bool[][])
                n349 = global write "自动测试结果.vi" "Auto_RS485_R"(w326) -> ()
                n350 = global write "自动测试结果.vi" "Auto_RS232_R"(w330) -> ()
                n351 = global write "自动测试结果.vi" "Auto_CAN_R"(w325) -> ()
                n352 = global write "自动测试结果.vi" "Auto_DSP_R"(w320) -> ()
                n353 = global write "自动测试结果.vi" "Auto_AD_R"(w322) -> ()
                n354 = global write "自动测试结果.vi" "Auto_DI_R"(w314) -> ()
                n355 = global write "自动测试结果.vi" "Auto_DO_R"(w318) -> ()
              }
              frame #6 {
                w332 = ""
                n356 = global read "试验配置信息.vi" "自测类数"() -> (w339:i32)
                n357 = global read "试验配置信息.vi" "自测项数"() -> (w336:i32)
                n358 = global read "试验配置信息.vi" "自测类数"() -> (w337:i32)
                n359 = global write "自动测试结果.vi" "数字量输入概述"(w332) -> ()
                n360 = global write "自动测试结果.vi" "数字量输出概述"(w332) -> ()
                n361 = global write "自动测试结果.vi" "模拟量DSP概述"(w332) -> ()
                n362 = global write "自动测试结果.vi" "模拟量AD概述结果"(w332) -> ()
                n363 = global write "自动测试结果.vi" "串口RS232测试概述"(w332) -> ()
                n364 = global write "自动测试结果.vi" "串口RS485测试概述"(w332) -> ()
                n365 = global write "自动测试结果.vi" "CAN测试概述"(w332) -> ()
                n366 = global write "自动测试结果.vi" "CAN测试概述"(w332) -> ()
                n367 = global write "自动测试结果.vi" "以太网测试概述"(w332) -> ()
                n368 = Divide(x=100, y=w339) -> (x/y=w341:dbl)
                n369 = property on="进度每次增加数" class="DigNum (严格)"("Value"=w341) -> ()  [unwired: 2 in, 2 out]
                n370 = Format Into String(format string="本报告测试项目共%d类，测试项总计%d项，其中：" ("时间格式字符串(%c)"), w337, w336) -> (resulting string=w334:string)  [unwired: 2 in, 1 out]
                n371 = Concatenate Strings(w334, "\r") -> (w335:string)
                n372 = global write "自动测试结果.vi" "自测总概述 temp"("") -> ()
                n373 = global write "自动测试结果.vi" "自测总概述"(w335) -> ()
              }
              frame #7 {
                w344 = "AutoStart" ("名称（未命名）")
                n374 = Obtain Notifier(name (unnamed)=w344, notification data type=w344) -> (notifier out=w343:refnum<notifier>)  [unwired: 2 in, 2 out]
                n375 = local write "进度提示"("正在测试中，请耐心等待结果......") -> ()
                n376 = Send Notification(notification="Auto" ("通知"), notifier=w343) -> ()  [unwired: 1 in, 2 out]
              }
              frame #8 {
                w346 = T3."Disabled and Grayed Out" ("禁用")
                n377 = property on="btn_数字输入" class="Bool"("DisabledEnum"=w346) -> ()  [unwired: 2 in, 2 out]
                n378 = property on="btn_数字输出" class="Bool"("DisabledEnum"=w346) -> ()  [unwired: 2 in, 2 out]
                n379 = property on="btn_DSP输入" class="Bool"("DisabledEnum"=w346) -> ()  [unwired: 2 in, 2 out]
                n380 = property on="btn_CAN总线" class="Bool"("DisabledEnum"=w346) -> ()  [unwired: 2 in, 2 out]
                n381 = property on="btn_R232_485总线" class="Bool"("DisabledEnum"=w346) -> ()  [unwired: 2 in, 2 out]
                n382 = property on="btn_LAN总线" class="Bool"("DisabledEnum"=w346) -> ()  [unwired: 2 in, 2 out]
                n383 = property on="函数类型 1" class="Bool"("DisabledEnum"=w346) -> ()  [unwired: 2 in, 2 out]
                n384 = property on="函数类型 2" class="Bool"("DisabledEnum"=w346) -> ()  [unwired: 2 in, 2 out]
                n385 = property on="函数类型 3" class="Bool"("DisabledEnum"=w346) -> ()  [unwired: 2 in, 2 out]
                n386 = property on="函数类型 4" class="Bool"("DisabledEnum"=w346) -> ()  [unwired: 2 in, 2 out]
                n387 = property on="btn_自动开始检测类型2" class="Bool"("DisabledEnum"=w346) -> ()  [unwired: 2 in, 2 out]
              }
            }
          }
        }
      }
      event "加载配置文件列表": Value Change {
        n388 = event-data() -> ()  [unwired: 1 in, 5 out]
        n389 = stacked-sequence {
          frame #0 {
            n390 = property on="加载配置文件列表" class="Ring (严格)"() -> ("RingText.Text"=w347:string)  [unwired: 2 in, 2 out]
            n391 = global write "试验配置信息.vi" "控制板类型"(w347) -> ()
          }
          frame #1 {
            # "判断 选择的是哪种类型板"
            n392 = local read "配置文件目录"() -> (w351:path)
            n393 = global read "试验配置信息.vi" "控制板类型"() -> (w352:string)
            n394 = call "罗列目录配置文件.vi"("路径"=w351) -> ("数组"=w349:string[])  [unwired: 10 in]
            n395 = Search 1D Array(1D array=w349, element=w352) -> (index of element=w353:i32)  [unwired: 1 in]
            n396 = Array Size(array=w349) -> (size(s)=w348:i32)
            n397 = Greater Or Equal To 0?(x=w353) -> (x >= 0?=w350:bool)
            n398 = case shown="假" w350 {
              tunnel: w348 -> [w355 _]
              frame False {
                n399 = local read "配置文件目录 2"() -> (w360:path)
                n400 = global write "试验配置信息.vi" "测试板卡类型"(enum16{"0", "1"}."1" ("测试板卡类型")) -> ()
                n401 = global read "试验配置信息.vi" "控制板类型"() -> (w359:string)
                n402 = call "罗列目录配置文件.vi"("路径"=w360) -> ("数组"=w358:string[])  [unwired: 10 in]
                n403 = Search 1D Array(1D array=w358, element=w359) -> (index of element=w357:i32)  [unwired: 1 in]
                n404 = Greater Or Equal To 0?(x=w357) -> (x >= 0?=w356:bool)
                n405 = case shown="真" w356 {
                  tunnel: w355 -> [_ w363]
                  frame False {
                  }
                  frame True {
                    n406 = property on="加载配置文件列表" class="Ring (严格)"() -> ("Value"=w361:u16)  [unwired: 2 in, 2 out]
                    n407 = property on="选项卡" class="TabCtl (严格)"("Value"=enum32{"板卡类型I", "板卡类型II"}."板卡类型II" ("选项卡")) -> ()  [unwired: 2 in, 2 out]
                    n408 = Subtract(x=w361, y=w363) -> (x-y=w362:i32)
                    n409 = global write "试验配置信息.vi" "文件序号"(w362) -> ()
                  }
                }
              }
              frame True {
                n410 = property on="选项卡" class="TabCtl (严格)"("Value"=enum32{"板卡类型I", "板卡类型II"}."板卡类型I" ("选项卡")) -> ()  [unwired: 2 in, 2 out]
                n411 = property on="加载配置文件列表" class="Ring (严格)"() -> ("Value"=w366:u16)  [unwired: 2 in, 2 out]
                n412 = global write "试验配置信息.vi" "测试板卡类型"(enum16{"0", "1"}."0" ("测试板卡类型")) -> ()
                n413 = global write "试验配置信息.vi" "文件序号"(w366) -> ()
              }
            }
          }
          frame #2 {
          }
          frame #3 {
            n414 = property on="选项卡" class="TabCtl (严格)"() -> ("Value"=w368:enum32{"板卡类型I", "板卡类型II"})  [unwired: 2 in, 2 out]
            n415 = case shown="\"板卡类型II\"" w368 {
              frame "板卡类型I", Default {
              }
              frame "板卡类型II" {
                n416 = local read "配置文件目录 2"() -> (w378:path)
                n417 = global read "试验配置信息.vi" "控制板类型"() -> (w379:string)
                n418 = Build Path(base path=w378, name or relative path=w379) -> (appended path=w377:path)
                n419 = call "函数测试配置文件读取.vi"("配置文件路径"=w377) -> ("类型1路数"=w372:i32, "类型2路数"=w371:i32, "类型3路数"=w370:i32, "类型4路数"=w369:i32, "D_IN_1"=w373:string[][], "D_IN_2"=w374:string[][], "D_IN_3"=w375:string[][], "D_IN_4"=w376:string[][])  [unwired: 11 in]
                n420 = global write "试验配置信息.vi" "D_IN_1"(w373) -> ()
                n421 = global write "试验配置信息.vi" "D_IN_2"(w374) -> ()
                n422 = global write "试验配置信息.vi" "D_IN_3"(w375) -> ()
                n423 = global write "试验配置信息.vi" "D_IN_4"(w376) -> ()
                n424 = global write "试验配置信息.vi" "自测类型4路数"(w369) -> ()
                n425 = global write "试验配置信息.vi" "自测类型3路数"(w370) -> ()
                n426 = global write "试验配置信息.vi" "自测类型2路数"(w371) -> ()
                n427 = global write "试验配置信息.vi" "自测类型1路数"(w372) -> ()
              }
            }
          }
          frame #4 {
            n428 = property on="选项卡" class="TabCtl (严格)"() -> ("Value"=w380:enum32{"板卡类型I", "板卡类型II"})  [unwired: 2 in, 2 out]
            n429 = case shown="\"板卡类型I\", 默认" w380 {
              frame "板卡类型I", Default {
                n430 = global read "试验配置信息.vi" "控制板类型"() -> (w390:string)
                n431 = call "读写配置文件.vi"("m_bCreat"=FALSE, "文件名称"=w390, "m_bRead"=TRUE) -> ("BoardConfig_output"=w391:T1)  [unwired: 8 in]
                n432 = global write "全局_配置.vi" "BoardConfig"(w391) -> ()
                n433 = Unbundle By Name(w391) -> ("数字量输入信号路数"=w388:i32, "数字量输出信号路数"=w387:i32, "DSP模拟量输入信号路数"=w386:u32, "DSP模拟量输入信号幅值"=w393:u32, "AD模拟量输入信号路数"=w385:u32, "AD模拟量输入信号幅值"=w396:u32, "RS232通信路数"=w384:u32, "RS232波特率"=w392:dbl, "RS485通信路数"=w383:u32, "CAN通信路数"=w382:i32)  [unwired: 7 out]
                n434 = case shown="0, 默认" w393 {
                  tunnel: [3.3 10.0 24.0] -> w394
                  frame 0, Default {
                  }
                  frame 1 {
                  }
                  frame 2 {
                  }
                }
                n435 = case shown="2" w396 {
                  tunnel: [6.0 10.0 24.0] -> w395
                  frame 0, Default {
                  }
                  frame 1 {
                  }
                  frame 2 {
                  }
                }
                n436 = global write "全局_配置.vi" "模拟量误差"(w392) -> ()
                n437 = global write "全局_配置.vi" "dsp模拟量输入路数"(w386) -> ()
                n438 = global write "全局_配置.vi" "数字量输出路数"(w387) -> ()
                n439 = global write "全局_配置.vi" "数字量输入路数"(w388) -> ()
                n440 = global write "全局_配置.vi" "ad模拟量输入路数"(w385) -> ()
                n441 = global write "试验配置信息.vi" "自测CAN路数"(w382) -> ()
                n442 = global write "全局_配置.vi" "R485路数"(w383) -> ()
                n443 = global write "全局_配置.vi" "R232路数"(w384) -> ()
                n444 = global write "全局_配置.vi" "DSP模拟量量程范围"(w394) -> ()
                n445 = global write "全局_配置.vi" "ARM模拟量量程范围"(w395) -> ()
              }
              frame "板卡类型II" {
              }
            }
          }
        }
      }
      event "btn_自动开始检测类型2": Value Change {
        w404 = ""
        n446 = event-data() -> ()  [unwired: 1 in, 5 out]
        n447 = local read "单选_函数类型1"() -> (w414:bool)
        n448 = local read "单选_函数类型2"() -> (w413:bool)
        n449 = local read "单选_函数类型3"() -> (w412:bool)
        n450 = local read "单选_函数类型4"() -> (w411:bool)
        n451 = local read "str_报告编号"() -> (w422:string)
        n452 = local read "str_测试编号"() -> (w421:string)
        n453 = local read "str_测试地点"() -> (w420:string)
        n454 = local read "str_测试人员"() -> (w419:string)
        n455 = property on="加载配置文件列表" class="Ring (严格)"() -> ("RingText.Text"=w405:string)  [unwired: 2 in, 2 out]
        n456 = Not Equal?(x=w405, y=w404) -> (x != y?=w403:bool)
        n457 = Not Equal?(x=w422, y=w404) -> (x != y?=w418:bool)
        n458 = Not Equal?(x=w421, y=w404) -> (x != y?=w417:bool)
        n459 = Not Equal?(x=w420, y=w404) -> (x != y?=w416:bool)
        n460 = Not Equal?(x=w419, y=w404) -> (x != y?=w415:bool)
        n461 = Compound Arithmetic op=AND(w403, w418, w417, w416, w415) -> (w409:bool)
        n462 = Compound Arithmetic op=OR(w414, w413, w412, w411) -> (w408:bool)
        n463 = And(x=w409, y=w408) -> (x .and. y?=w410:bool)
        n464 = case shown="真" w410 {
          tunnel: w409 -> [w424 _]
          tunnel: w408 -> [w423 _]
          tunnel: w407 -> [_ w426]
          tunnel: w406 -> [_ w425]
          frame False {
            n465 = case shown="假" w424 {
              frame False {
                n466 = call "显示对话框信息3"() -> ()  [unwired: 10 in, 2 out]
              }
              frame True {
              }
            }
            n467 = case shown="假" w423 {
              frame False {
                n468 = call "显示对话框信息4"() -> ()  [unwired: 10 in, 2 out]
              }
              frame True {
              }
            }
          }
          frame True {
            n469 = stacked-sequence {
              tunnel: w426 -> [_ _ _ _ _ _ w531 _]
              tunnel: w425 -> [_ _ _ _ _ _ w530 _]
              frame #0 {
                n470 = property on="加载配置文件列表" class="Ring (严格)"() -> ("RingText.Text"=w432:string)  [unwired: 2 in, 2 out]
                n471 = local read "str_测试人员"() -> (w430:string)
                n472 = local read "str_报告编号"() -> (w436:string)
                n473 = local read "str_测试编号"() -> (w437:string)
                n474 = local read "str_测试地点"() -> (w439:string)
                n475 = local read "str_测试人员"() -> (w438:string)
                n476 = local read "str_测试地点"() -> (w429:string)
                n477 = local read "str_报告编号"() -> (w434:string)
                n478 = local read "str_测试编号"() -> (w433:string)
                n479 = global write "试验配置信息.vi" "报告编号"(w436) -> ()
                n480 = global write "试验配置信息.vi" "控制板编号"(w437) -> ()
                n481 = global write "试验配置信息.vi" "测试地点"(w439) -> ()
                n482 = global write "试验配置信息.vi" "测试人员"(w438) -> ()
                n483 = Bundle("str_报告编号"=w434, "str_测试编号"=w433, "RingText.Text"=w432, "str_测试人员"=w430, "str_测试地点"=w429) -> (w431:T2)  [unwired: 1 in]
                n484 = global write "试验配置信息.vi" "控制板类型"(w432) -> ()
                n485 = global write "试验配置信息.vi" "自测类数"(0 ("自测类数")) -> ()
                n486 = global write "试验配置信息.vi" "自测项数"(0 ("自测类数")) -> ()
                n487 = call "实验配置信息读取和写入.vi"("读取写入"=TRUE, "输入簇"=w431) -> ()  [unwired: 7 in, 1 out]
              }
              frame #1 {
                n488 = stacked-sequence {
                  frame #0 {
                    n489 = global read "试验配置信息.vi" "D_IN_1"() -> (w446:string[][])
                    n490 = global read "试验配置信息.vi" "自测类型1路数"() -> (w447:i32)
                    n491 = Index Array(array=w446, index (row)=0 ("索引"), index (col)=1 ("禁用的索引 (列)")) -> (element=w443:string)
                    n492 = local read "单选_函数类型1"() -> (w448:bool)
                    n493 = String Length(string=w443) -> (length=w442:i32)
                    n494 = Greater Than 0?(x=w447) -> (x > 0?=w441:bool)
                    n495 = Greater Than 0?(x=w442) -> (x > 0?=w440:bool)
                    n496 = Compound Arithmetic op=AND(w448, w441, w440) -> (w449:bool)
                    n497 = global write "试验配置信息.vi" "测试类型1选择？"(w449) -> ()
                  }
                  frame #1 {
                    n498 = global read "试验配置信息.vi" "D_IN_2"() -> (w456:string[][])
                    n499 = global read "试验配置信息.vi" "自测类型2路数"() -> (w457:i32)
                    n500 = Index Array(array=w456, index (row)=0 ("索引"), index (col)=1 ("禁用的索引 (列)")) -> (element=w453:string)
                    n501 = local read "单选_函数类型2"() -> (w458:bool)
                    n502 = String Length(string=w453) -> (length=w452:i32)
                    n503 = Greater Than 0?(x=w457) -> (x > 0?=w451:bool)
                    n504 = Greater Than 0?(x=w452) -> (x > 0?=w450:bool)
                    n505 = Compound Arithmetic op=AND(w458, w451, w450) -> (w459:bool)
                    n506 = global write "试验配置信息.vi" "测试类型2选择？"(w459) -> ()
                  }
                  frame #2 {
                    n507 = global read "试验配置信息.vi" "D_IN_3"() -> (w466:string[][])
                    n508 = global read "试验配置信息.vi" "自测类型3路数"() -> (w467:i32)
                    n509 = Index Array(array=w466, index (row)=0 ("索引"), index (col)=1 ("禁用的索引 (列)")) -> (element=w463:string)
                    n510 = local read "单选_函数类型3"() -> (w468:bool)
                    n511 = String Length(string=w463) -> (length=w462:i32)
                    n512 = Greater Than 0?(x=w467) -> (x > 0?=w461:bool)
                    n513 = Greater Than 0?(x=w462) -> (x > 0?=w460:bool)
                    n514 = Compound Arithmetic op=AND(w468, w461, w460) -> (w469:bool)
                    n515 = global write "试验配置信息.vi" "测试类型3选择？"(w469) -> ()
                  }
                  frame #3 {
                    n516 = global read "试验配置信息.vi" "D_IN_4"() -> (w476:string[][])
                    n517 = global read "试验配置信息.vi" "自测类型4路数"() -> (w477:i32)
                    n518 = Index Array(array=w476, index (row)=0 ("索引"), index (col)=1 ("禁用的索引 (列)")) -> (element=w473:string)
                    n519 = local read "单选_函数类型4"() -> (w478:bool)
                    n520 = String Length(string=w473) -> (length=w472:i32)
                    n521 = Greater Than 0?(x=w477) -> (x > 0?=w471:bool)
                    n522 = Greater Than 0?(x=w472) -> (x > 0?=w470:bool)
                    n523 = Compound Arithmetic op=AND(w478, w471, w470) -> (w479:bool)
                    n524 = global write "试验配置信息.vi" "测试类型4选择？"(w479) -> ()
                  }
                }
              }
              frame #2 {
                n525 = global read "试验配置信息.vi" "测试类型1选择？"() -> (w483:bool)
                n526 = global read "试验配置信息.vi" "测试类型2选择？"() -> (w482:bool)
                n527 = global read "试验配置信息.vi" "测试类型3选择？"() -> (w481:bool)
                n528 = global read "试验配置信息.vi" "测试类型4选择？"() -> (w480:bool)
                n529 = Build Array(w483, w482, w481, w480) -> (w484:bool[])
                n530 = for {
                  tunnel: w484 -> [w485] mode=indexing
                  n531 = case shown="真" w485 {
                    frame False {
                    }
                    frame True {
                      n532 = global read "试验配置信息.vi" "自测类数"() -> (w487:i32)
                      n533 = Increment(x=w487) -> (x+1=w486:i32)
                      n534 = global write "试验配置信息.vi" "自测类数"(w486) -> ()
                    }
                  }
                }
              }
              frame #3 {
                n535 = global read "试验配置信息.vi" "测试类型1选择？"() -> (w496:bool)
                n536 = global read "试验配置信息.vi" "测试类型2选择？"() -> (w495:bool)
                n537 = global read "试验配置信息.vi" "测试类型3选择？"() -> (w494:bool)
                n538 = global read "试验配置信息.vi" "测试类型4选择？"() -> (w493:bool)
                n539 = case shown="真" w496 {
                  tunnel: [0 w504] -> w492
                  frame False {
                  }
                  frame True {
                    n540 = global read "试验配置信息.vi" "自测类型1路数"() -> (w504:i32)
                  }
                }
                n541 = case shown="真" w494 {
                  tunnel: [0 w500] -> w490
                  frame False {
                  }
                  frame True {
                    n542 = global read "试验配置信息.vi" "自测类型3路数"() -> (w500:i32)
                  }
                }
                n543 = case shown="真" w495 {
                  tunnel: [0 w502] -> w491
                  frame False {
                  }
                  frame True {
                    n544 = global read "试验配置信息.vi" "自测类型2路数"() -> (w502:i32)
                  }
                }
                n545 = case shown="真" w493 {
                  tunnel: [0 w498] -> w489
                  frame False {
                  }
                  frame True {
                    n546 = global read "试验配置信息.vi" "自测类型4路数"() -> (w498:i32)
                  }
                }
                n547 = Compound Arithmetic op=ADD(w492, w491, w490, w489) -> (w488:i32)
                n548 = global write "试验配置信息.vi" "自测项数"(w488) -> ()
              }
              frame #4 {
                n549 = global read "试验配置信息.vi" "自测类型1路数"() -> (w509:i32)
                n550 = global read "试验配置信息.vi" "自测类型2路数"() -> (w512:i32)
                n551 = global read "试验配置信息.vi" "自测类型3路数"() -> (w515:i32)
                n552 = global read "试验配置信息.vi" "自测类型4路数"() -> (w518:i32)
                n553 = global read "试验配置信息.vi" "自测类型1路数"() -> (w505:i32)
                n554 = Initialize Array(TRUE ("元素"), w509) -> (w508:bool[])
                n555 = Initialize Array(TRUE ("元素"), w512) -> (w513:bool[])
                n556 = Initialize Array(TRUE ("元素"), w515) -> (w514:bool[])
                n557 = Initialize Array(TRUE ("元素"), w518) -> (w519:bool[])
                n558 = Initialize Array(0.0, w505) -> (w507:dbl[])
                n559 = global write "自动测试结果.vi" "Auto_func_1_R"(w508) -> ()
                n560 = global write "自动测试结果.vi" "Auto_func_2_R"(w513) -> ()
                n561 = global write "自动测试结果.vi" "Auto_func_3_R"(w514) -> ()
                n562 = global write "自动测试结果.vi" "Auto_func_4_R"(w519) -> ()
                n563 = global write "自动测试结果.vi" "Auto_func_1_max_WC"(w507) -> ()
              }
              frame #5 {
                w522 = string[][] [["序号", "测试项", "输出通道", "输入通道", "测试结果"]] ("自动测试结果")
                w520 = string[][] [["序号", "测试项", "输出通道", "输入通道试结果", "最大误差(%)", "测试结果"]] ("自动测试结果")
                w523 = ""
                n564 = global read "试验配置信息.vi" "自测项数"() -> (w527:i32)
                n565 = global read "试验配置信息.vi" "自测类数"() -> (w528:i32)
                n566 = global write "自动测试结果.vi" "测试类型1概述"(w523) -> ()
                n567 = global write "自动测试结果.vi" "测试类型2概述"(w523) -> ()
                n568 = global write "自动测试结果.vi" "测试类型3概述"(w523) -> ()
                n569 = global write "自动测试结果.vi" "测试类型4概述"(w523) -> ()
                n570 = Format Into String(format string="本报告测试项目共%d类，测试项总计%d项，其中：" ("时间格式字符串(%c)"), w528, w527) -> (resulting string=w525:string)  [unwired: 2 in, 1 out]
                n571 = global write "自动测试结果.vi" "测试类型1自动测试结果"(w520) -> ()
                n572 = global write "自动测试结果.vi" "测试类型2自动测试结果"(w520) -> ()
                n573 = global write "自动测试结果.vi" "测试类型3自动测试结果"(w522) -> ()
                n574 = global write "自动测试结果.vi" "测试类型4自动测试结果"(w522) -> ()
                n575 = Concatenate Strings(w525, "\r") -> (w526:string)
                n576 = global write "自动测试结果.vi" "自测总概述 temp"("") -> ()
                n577 = global write "自动测试结果.vi" "自测总概述"(w526) -> ()
              }
              frame #6 {
                n578 = local write "进度提示"("正在测试中，请耐心等待结果......") -> ()
                n579 = Send Notification(notification="Auto_2" ("通知"), notifier=w531, error in (no error)=w530) -> ()  [unwired: 2 out]
              }
              frame #7 {
                w534 = T3."Disabled and Grayed Out" ("禁用")
                n580 = property on="btn_数字输入" class="Bool"("DisabledEnum"=w534) -> ()  [unwired: 2 in, 2 out]
                n581 = property on="btn_数字输出" class="Bool"("DisabledEnum"=w534) -> ()  [unwired: 2 in, 2 out]
                n582 = property on="btn_DSP输入" class="Bool"("DisabledEnum"=w534) -> ()  [unwired: 2 in, 2 out]
                n583 = property on="btn_CAN总线" class="Bool"("DisabledEnum"=w534) -> ()  [unwired: 2 in, 2 out]
                n584 = property on="btn_R232_485总线" class="Bool"("DisabledEnum"=w534) -> ()  [unwired: 2 in, 2 out]
                n585 = property on="btn_LAN总线" class="Bool"("DisabledEnum"=w534) -> ()  [unwired: 2 in, 2 out]
                n586 = property on="函数类型 1" class="Bool"("DisabledEnum"=w534) -> ()  [unwired: 2 in, 2 out]
                n587 = property on="函数类型 2" class="Bool"("DisabledEnum"=w534) -> ()  [unwired: 2 in, 2 out]
                n588 = property on="函数类型 3" class="Bool"("DisabledEnum"=w534) -> ()  [unwired: 2 in, 2 out]
                n589 = property on="函数类型 4" class="Bool"("DisabledEnum"=w534) -> ()  [unwired: 2 in, 2 out]
                n590 = property on="btn_开始检测" class="Bool"("DisabledEnum"=w534) -> ()  [unwired: 2 in, 2 out]
              }
            }
          }
        }
      }
      event "单选_函数类型1": Value Change {
        n591 = event-data() -> ("NewVal"=w535:bool)  [unwired: 1 in, 4 out]
        n592 = local write "单选_函数类型1"(w535) -> ()
      }
      event "单选_函数类型2": Value Change {
        n593 = event-data() -> ("NewVal"=w536:bool)  [unwired: 1 in, 4 out]
        n594 = local write "单选_函数类型2"(w536) -> ()
      }
      event "单选_函数类型3": Value Change {
        n595 = event-data() -> ("NewVal"=w537:bool)  [unwired: 1 in, 4 out]
        n596 = local write "单选_函数类型3"(w537) -> ()
      }
      event "单选_函数类型4": Value Change {
        n597 = event-data() -> ("NewVal"=w538:bool)  [unwired: 1 in, 4 out]
        n598 = local write "单选_函数类型4"(w538) -> ()
      }
      event "通道及参数配置": Value Change {
        n599 = event-data() -> ()  [unwired: 1 in, 5 out]
        n600 = stacked-sequence {
          frame #0 {
          }
          frame #1 {
            n601 = call "通道配置模块.vi"() -> ("返回"=w539:bool)  [unwired: 11 in]
            n602 = case shown="真" w539 {
              frame False {
              }
              frame True {
                n603 = stacked-sequence {
                  frame #0 {
                    # "遍历配置文件目录"
                    n604 = local read "配置文件目录"() -> (w544:path)
                    n605 = local read "配置文件目录 2"() -> (w543:path)
                    n606 = call "罗列目录配置文件.vi"("路径"=w544) -> ("数组"=w542:string[])  [unwired: 10 in]
                    n607 = call "罗列目录配置文件.vi"("路径"=w543) -> ("数组"=w541:string[])  [unwired: 10 in]
                    n608 = Insert Into Array(array=w542, new element=w541) -> (w540:string[])  [unwired: 1 in]
                    n609 = property on="加载配置文件列表" class="Ring (严格)"("Strings []"=w540) -> ()  [unwired: 2 in, 2 out]
                  }
                  frame #1 {
                    n610 = global read "试验配置信息.vi" "测试板卡类型"() -> (w545:enum16{"0", "1"})
                    n611 = case shown="\"1\"" w545 {
                      frame "0", Default {
                        n612 = property on="选项卡" class="TabCtl (严格)"("Value"=0) -> ()  [unwired: 2 in, 2 out]
                        n613 = global read "试验配置信息.vi" "文件序号"() -> (w546:i32)
                        n614 = property on="加载配置文件列表" class="Ring (严格)"("Value"=w546) -> ()  [unwired: 2 in, 2 out]
                      }
                      frame "1" {
                        # "遍历配置文件目录"
                        n615 = local read "配置文件目录"() -> (w552:path)
                        n616 = property on="选项卡" class="TabCtl (严格)"("Value"=1) -> ()  [unwired: 2 in, 2 out]
                        n617 = global read "试验配置信息.vi" "文件序号"() -> (w550:i32)
                        n618 = call "罗列目录配置文件.vi"("路径"=w552) -> ("数组"=w551:string[])  [unwired: 10 in]
                        n619 = Array Size(array=w551) -> (size(s)=w549:i32)
                        n620 = Add(x=w550, y=w549) -> (x+y=w548:i32)
                        n621 = property on="加载配置文件列表" class="Ring (严格)"("Value"=w548) -> ()  [unwired: 2 in, 2 out]
                      }
                    }
                  }
                }
              }
            }
          }
        }
      }
      event "函数类型 1": Value Change {
        n622 = event-data() -> ()  [unwired: 1 in, 5 out]
        n623 = call "函数类型1测试.vi"() -> ()  [unwired: 12 in]
      }
      event "btn_二维码识别": Value Change {
        n624 = event-data() -> ()  [unwired: 1 in, 5 out]
        n625 = stacked-sequence {
          frame #0 {
            n626 = local read "str_测试编号"() -> (w554:string)
            n627 = global write "试验配置信息.vi" "条形码"(w554) -> ()
          }
          frame #1 {
            n628 = call "生成板卡编号.vi"() -> ("bCreate"=w555:bool)  [unwired: 11 in]
            n629 = case shown="真" w555 {
              frame False {
              }
              frame True {
                n630 = global read "试验配置信息.vi" "条形码"() -> (w556:string)
                n631 = local write "str_测试编号"(w556) -> ()
              }
            }
          }
        }
      }
      event "函数类型 1": Mouse Leave {
        n632 = event-data() -> ()  [unwired: 1 in, 3 out]
        n633 = property on="函数类型 1" class="Bool"("Caption.Visible"=FALSE ("标签.可见")) -> ()  [unwired: 2 in, 2 out]
      }
      event "函数类型 1": Mouse Enter {
        n634 = event-data() -> ()  [unwired: 1 in, 3 out]
        n635 = property on="函数类型 1" class="Bool"("Caption.Visible"=TRUE ("标签.可见")) -> ()  [unwired: 2 in, 2 out]
      }
      event "函数类型 2": Value Change {
        n636 = event-data() -> ()  [unwired: 1 in, 5 out]
        n637 = call "函数类型2测试.vi"() -> ()  [unwired: 12 in]
      }
      event "函数类型 2": Mouse Enter {
        n638 = event-data() -> ()  [unwired: 1 in, 3 out]
        n639 = property on="函数类型 2" class="Bool"("Caption.Visible"=TRUE) -> ()  [unwired: 2 in, 2 out]
      }
      event "函数类型 2": Mouse Leave {
        n640 = event-data() -> ()  [unwired: 1 in, 3 out]
        n641 = property on="函数类型 2" class="Bool"("Caption.Visible"=FALSE) -> ()  [unwired: 2 in, 2 out]
      }
      event "函数类型 3": Value Change {
        n642 = event-data() -> ()  [unwired: 1 in, 5 out]
        n643 = call "函数类型3测试.vi"() -> ()  [unwired: 12 in]
      }
      event "函数类型 3": Mouse Enter {
        n644 = event-data() -> ()  [unwired: 1 in, 3 out]
        n645 = property on="函数类型 3" class="Bool"("Caption.Visible"=TRUE) -> ()  [unwired: 2 in, 2 out]
      }
      event "函数类型 3": Mouse Leave {
        n646 = event-data() -> ()  [unwired: 1 in, 3 out]
        n647 = property on="函数类型 3" class="Bool"("Caption.Visible"=FALSE) -> ()  [unwired: 2 in, 2 out]
      }
      event "函数类型 4": Value Change {
        n648 = event-data() -> ()  [unwired: 1 in, 5 out]
        n649 = call "函数类型4测试.vi"() -> ()  [unwired: 12 in]
      }
      event "函数类型 4": Mouse Enter {
        n650 = event-data() -> ()  [unwired: 1 in, 3 out]
        n651 = property on="函数类型 4" class="Bool"("Caption.Visible"=TRUE) -> ()  [unwired: 2 in, 2 out]
      }
      event "函数类型 4": Mouse Leave {
        n652 = event-data() -> ()  [unwired: 1 in, 3 out]
        n653 = property on="函数类型 4" class="Bool"("Caption.Visible"=FALSE) -> ()  [unwired: 2 in, 2 out]
      }
    }
    n654 = local write "退出？"(w179) -> ()
    n655 = Quit LabVIEW(quit? (T)=w179) -> ()
  }
  n656 = Obtain Notifier(name (unnamed)=w14, notification data type=w14) -> (notifier out=w13:refnum<notifier>, error out=w12:errorcluster)  [unwired: 2 in, 1 out]
  n657 = while {
    tunnel: w13 -> [w574]
    tunnel: w12 -> [w573]
    tunnel: [w572] -> w11
    tunnel: [w571] -> w10
    stop <- w566 stop-if-true
    # "I型板自动测试"
    n658 = Wait Until Next ms Multiple(millisecond multiple=u32 20 ("毫秒倍数")) -> ()  [unwired: 1 out]
    n659 = Wait on Notification(notifier=w574, timeout in ms (-1)=20 ("超时毫秒(-1)"), error in (no error)=w573) -> (notifier out=w572:refnum<notifier>, notification=w569:string, error out=w571:errorcluster)  [unwired: 1 in, 1 out]
    n660 = Equal?(x=w569, y="Auto" ("通知")) -> (x = y?=w568:bool)
    n661 = case shown="真" w568 {
      frame False {
      }
      frame True {
        n662 = stacked-sequence {
          frame #0 {
            n663 = global read "试验配置信息.vi" "数字量输入选择？"() -> (w575:bool)
            n664 = case shown="真" w575 {
              frame False {
              }
              frame True {
                # "数字量输入"
                n665 = local read "单选_数字量输入"() -> (w576:bool)
                n666 = stacked-sequence {
                  tunnel: w576 -> [w578 w579]
                  frame #0 {
                    n667 = call "数字量输入自动检测.vi"("选择?"=w578) -> ()  [unwired: 11 in]
                    n668 = local write "进度提示"("正在进行数字量输入测试......") -> ()
                  }
                  frame #1 {
                    n669 = case shown="真" w579 {
                      frame False {
                      }
                      frame True {
                        n670 = global read "试验配置信息.vi" "自动检测结果"() -> (w581:bool[])
                        n671 = Index Array(array=w581, index=0) -> (element=w583:bool)
                        n672 = case shown="真" w583 {
                          tunnel: [2 1] -> w584
                          frame False {
                          }
                          frame True {
                          }
                        }
                        n673 = case shown="0, 默认" w584 {
                          tunnel: [cluster{u32, u32}[] [{1985280, 1985280}] cluster{u32, u32}[] [{61205, 6618880}] cluster{u32, u32}[] [{16730410, 16711680}]] -> w580
                          frame 0, Default {
                          }
                          frame 1 {
                          }
                          frame 2 {
                          }
                        }
                        n674 = property on="数字量输入检测" class="Bool (严格)"("Colors [4]"=w580) -> ()  [unwired: 2 in, 2 out]
                      }
                    }
                  }
                }
              }
            }
          }
          frame #1 {
            n675 = global read "试验配置信息.vi" "数字量输出选择？"() -> (w590:bool)
            n676 = case shown="真" w590 {
              frame False {
              }
              frame True {
                # "数字量输出"
                n677 = local read "单选_数字量输出"() -> (w591:bool)
                n678 = stacked-sequence {
                  tunnel: w591 -> [w593 w594]
                  frame #0 {
                    n679 = call "自动数量输出.vi"("选择？"=w593) -> ()  [unwired: 11 in]
                    n680 = local write "进度提示"("正在进行数字量输出测试......") -> ()
                  }
                  frame #1 {
                    n681 = case shown="真" w594 {
                      frame False {
                      }
                      frame True {
                        n682 = global read "试验配置信息.vi" "自动检测结果"() -> (w596:bool[])
                        n683 = Index Array(array=w596, index=1) -> (element=w598:bool)
                        n684 = case shown="假" w598 {
                          tunnel: [2 1] -> w599
                          frame False {
                          }
                          frame True {
                          }
                        }
                        n685 = case shown="0, 默认" w599 {
                          tunnel: [cluster{u32, u32}[] [{1985280, 1985280}] cluster{u32, u32}[] [{61205, 6618880}] cluster{u32, u32}[] [{16730410, 16711680}]] -> w595
                          frame 0, Default {
                          }
                          frame 1 {
                          }
                          frame 2 {
                          }
                        }
                        n686 = property on="数字量输出检测" class="Bool (严格)"("Colors [4]"=w595) -> ()  [unwired: 2 in, 2 out]
                      }
                    }
                  }
                }
              }
            }
          }
          frame #2 {
            # "模拟量输入"
            n687 = global read "试验配置信息.vi" "DSP输入选择？"() -> (w605:bool)
            n688 = global read "试验配置信息.vi" "AD输入选择？"() -> (w606:bool)
            n689 = stacked-sequence {
              tunnel: w605 -> [w609 w611]
              tunnel: w606 -> [w608 w610]
              frame #0 {
                n690 = call "模拟量输入自动测试.vi"("AD选择?"=w608, "DSP选择?"=w609) -> ()  [unwired: 10 in]
                n691 = local write "进度提示"("正在进行模拟量测试......") -> ()
              }
              frame #1 {
                n692 = stacked-sequence {
                  tunnel: w611 -> [w612 _]
                  tunnel: w610 -> [_ w623]
                  frame #0 {
                    n693 = case shown="真" w612 {
                      frame False {
                      }
                      frame True {
                        n694 = global read "试验配置信息.vi" "自动检测结果"() -> (w614:bool[])
                        n695 = Index Array(array=w614, index=2) -> (element=w616:bool)
                        n696 = case shown="假" w616 {
                          tunnel: [2 1] -> w617
                          frame False {
                          }
                          frame True {
                          }
                        }
                        n697 = case shown="0, 默认" w617 {
                          tunnel: [cluster{u32, u32}[] [{1985280, 1985280}] cluster{u32, u32}[] [{61205, 6618880}] cluster{u32, u32}[] [{16730410, 16711680}]] -> w613
                          frame 0, Default {
                          }
                          frame 1 {
                          }
                          frame 2 {
                          }
                        }
                        n698 = property on="模拟量DSP输入检测" class="Bool (严格)"("Colors [4]"=w613) -> ()  [unwired: 2 in, 2 out]
                      }
                    }
                  }
                  frame #1 {
                    n699 = case shown="真" w623 {
                      frame False {
                      }
                      frame True {
                        n700 = global read "试验配置信息.vi" "自动检测结果"() -> (w625:bool[])
                        n701 = Index Array(array=w625, index=3) -> (element=w627:bool)
                        n702 = case shown="假" w627 {
                          tunnel: [2 1] -> w628
                          frame False {
                          }
                          frame True {
                          }
                        }
                        n703 = case shown="2" w628 {
                          tunnel: [cluster{u32, u32}[] [{1985280, 1985280}] cluster{u32, u32}[] [{61205, 6618880}] cluster{u32, u32}[] [{16730410, 16711680}]] -> w624
                          frame 0, Default {
                          }
                          frame 1 {
                          }
                          frame 2 {
                          }
                        }
                        n704 = property on="模拟量AD输入检测" class="Bool (严格)"("Colors [4]"=w624) -> ()  [unwired: 2 in, 2 out]
                      }
                    }
                  }
                }
              }
            }
          }
          frame #3 {
            n705 = global read "试验配置信息.vi" "RS485选择？"() -> (w634:bool)
            n706 = global read "试验配置信息.vi" "RS232选择？"() -> (w635:bool)
            n707 = stacked-sequence {
              tunnel: w635 -> [w638 w640]
              tunnel: w634 -> [w637 w639]
              frame #0 {
                n708 = call "串口自动测试.vi"("RS485选择"=w637, "RS232选择"=w638) -> ()  [unwired: 10 in]
                n709 = local write "进度提示"("正在进行串口测试......") -> ()
              }
              frame #1 {
                n710 = stacked-sequence {
                  tunnel: w640 -> [w641 _]
                  tunnel: w639 -> [_ w652]
                  frame #0 {
                    n711 = case shown="真" w641 {
                      frame False {
                      }
                      frame True {
                        n712 = global read "试验配置信息.vi" "自动检测结果"() -> (w643:bool[])
                        n713 = Index Array(array=w643, index=4) -> (element=w645:bool)
                        n714 = case shown="假" w645 {
                          tunnel: [2 1] -> w646
                          frame False {
                          }
                          frame True {
                          }
                        }
                        n715 = case shown="0, 默认" w646 {
                          tunnel: [cluster{u32, u32}[] [{1985280, 1985280}] cluster{u32, u32}[] [{61205, 6618880}] cluster{u32, u32}[] [{16730410, 16711680}]] -> w642
                          frame 0, Default {
                          }
                          frame 1 {
                          }
                          frame 2 {
                          }
                        }
                        n716 = property on="RS232总线检测" class="Bool (严格)"("Colors [4]"=w642) -> ()  [unwired: 2 in, 2 out]
                      }
                    }
                  }
                  frame #1 {
                    n717 = case shown="真" w652 {
                      frame False {
                      }
                      frame True {
                        n718 = global read "试验配置信息.vi" "自动检测结果"() -> (w654:bool[])
                        n719 = Index Array(array=w654, index=5) -> (element=w656:bool)
                        n720 = case shown="假" w656 {
                          tunnel: [2 1] -> w657
                          frame False {
                          }
                          frame True {
                          }
                        }
                        n721 = case shown="0, 默认" w657 {
                          tunnel: [cluster{u32, u32}[] [{1985280, 1985280}] cluster{u32, u32}[] [{61205, 6618880}] cluster{u32, u32}[] [{16730410, 16711680}]] -> w653
                          frame 0, Default {
                          }
                          frame 1 {
                          }
                          frame 2 {
                          }
                        }
                        n722 = property on="RS485总线检测" class="Bool (严格)"("Colors [4]"=w653) -> ()  [unwired: 2 in, 2 out]
                      }
                    }
                  }
                }
              }
            }
          }
          frame #4 {
            n723 = global read "试验配置信息.vi" "CAN选择？"() -> (w663:bool)
            n724 = stacked-sequence {
              tunnel: w663 -> [w665 w666]
              frame #0 {
                n725 = call "CAN自动测试.vi"("选择?"=w665) -> ()  [unwired: 11 in]
                n726 = local write "进度提示"("正在进行CAN测试......") -> ()
              }
              frame #1 {
                n727 = case shown="真" w666 {
                  frame False {
                  }
                  frame True {
                    n728 = global read "试验配置信息.vi" "自动检测结果"() -> (w668:bool[])
                    n729 = Index Array(array=w668, index=6) -> (element=w670:bool)
                    n730 = case shown="假" w670 {
                      tunnel: [2 1] -> w671
                      frame False {
                      }
                      frame True {
                      }
                    }
                    n731 = case shown="0, 默认" w671 {
                      tunnel: [cluster{u32, u32}[] [{1985280, 1985280}] cluster{u32, u32}[] [{61205, 6618880}] cluster{u32, u32}[] [{16730410, 16711680}]] -> w667
                      frame 0, Default {
                      }
                      frame 1 {
                      }
                      frame 2 {
                      }
                    }
                    n732 = property on="CAN总线检测" class="Bool (严格)"("Colors [4]"=w667) -> ()  [unwired: 2 in, 2 out]
                  }
                }
              }
            }
          }
          frame #5 {
            # "以太网"
            n733 = local read "单选_LAN检测"() -> (w677:bool)
            n734 = case shown="真" w677 {
              tunnel: w677 -> [_ w678]
              frame False {
              }
              frame True {
                n735 = stacked-sequence {
                  tunnel: w678 -> [w680 w681]
                  frame #0 {
                    n736 = call "以太网自动测试.vi"("选择?"=w680) -> ()  [unwired: 11 in]
                    n737 = local write "进度提示"("正在进行LAN测试......") -> ()
                  }
                  frame #1 {
                    n738 = case shown="真" w681 {
                      frame False {
                      }
                      frame True {
                        n739 = global read "试验配置信息.vi" "自动检测结果"() -> (w683:bool[])
                        n740 = Index Array(array=w683, index=7) -> (element=w685:bool)
                        n741 = case shown="假" w685 {
                          tunnel: [2 1] -> w686
                          frame False {
                          }
                          frame True {
                          }
                        }
                        n742 = case shown="0, 默认" w686 {
                          tunnel: [cluster{u32, u32}[] [{1985280, 1985280}] cluster{u32, u32}[] [{61205, 6618880}] cluster{u32, u32}[] [{16730410, 16711680}]] -> w682
                          frame 0, Default {
                          }
                          frame 1 {
                          }
                          frame 2 {
                          }
                        }
                        n743 = property on="LAN总线检测" class="Bool (严格)"("Colors [4]"=w682) -> ()  [unwired: 2 in, 2 out]
                      }
                    }
                  }
                }
              }
            }
          }
          frame #6 {
            # "统计合格率"
            n744 = call "统计合格率.vi"() -> ()  [unwired: 12 in]
          }
          frame #7 {
            n745 = flat-sequence {
              tunnel: [w693] -> w692
              tunnel: w692 -> [w696]
              frame #0 {
                # "报告存储"
                n746 = Get Date/Time In Seconds() -> (seconds since 1Jan1904=w693:timestamp)
                n747 = call "报告存储.vi"("生成报告?"=FALSE, "是否存储到数据库?"=TRUE, "试验时间"=w693) -> ()  [unwired: 9 in]
              }
              frame #1 {
                n748 = global read "自动测试结果.vi" "自测总概述 temp"() -> (w698:string)
                n749 = call "完成"("Message"=w698) -> ("生成报告"=w697:bool)  [unwired: 9 in, 1 out]
                n750 = case shown="真" w697 {
                  tunnel: w696 -> [_ w701]
                  frame False {
                  }
                  frame True {
                    n751 = call "报告存储.vi"("生成报告?"=TRUE, "是否存储到数据库?"=FALSE, "试验时间"=w701) -> ()  [unwired: 9 in]
                  }
                }
              }
            }
            n752 = disable-structure shown="禁用" {
              frame Disabled {
                n753 = Get Date/Time In Seconds() -> (seconds since 1Jan1904=w702:timestamp)
                n754 = call "测试报告摘要4.vi"("打印?"=FALSE, "试验时间"=w702) -> ()  [unwired: 10 in]
              }
              frame Enabled {
              }
            }
          }
          frame #8 {
            w705 = T3."Enabled" ("禁用")
            n755 = case shown="0, 默认" 0 {
              tunnel: [cluster{u32, u32}[] [{1985280, 1985280}] cluster{u32, u32}[] [{61205, 6618880}] cluster{u32, u32}[] [{16730410, 16711680}]] -> w706
              frame 0, Default {
              }
              frame 1 {
              }
              frame 2 {
              }
            }
            n756 = property on="数字量输入检测" class="Bool (严格)"("Colors [4]"=w706) -> ()  [unwired: 2 in, 2 out]
            n757 = property on="数字量输出检测" class="Bool (严格)"("Colors [4]"=w706) -> ()  [unwired: 2 in, 2 out]
            n758 = property on="模拟量AD输入检测" class="Bool (严格)"("Colors [4]"=w706) -> ()  [unwired: 2 in, 2 out]
            n759 = property on="CAN总线检测" class="Bool (严格)"("Colors [4]"=w706) -> ()  [unwired: 2 in, 2 out]
            n760 = local write "进度提示"("测试完毕......") -> ()
            n761 = property on="LAN总线检测" class="Bool (严格)"("Colors [4]"=w706) -> ()  [unwired: 2 in, 2 out]
            n762 = property on="RS232总线检测" class="Bool (严格)"("Colors [4]"=w706) -> ()  [unwired: 2 in, 2 out]
            n763 = property on="RS485总线检测" class="Bool (严格)"("Colors [4]"=w706) -> ()  [unwired: 2 in, 2 out]
            n764 = property on="模拟量DSP输入检测" class="Bool (严格)"("Colors [4]"=w706) -> ()  [unwired: 2 in, 2 out]
            n765 = property on="btn_数字输入" class="Bool"("DisabledEnum"=w705) -> ()  [unwired: 2 in, 2 out]
            n766 = property on="btn_数字输出" class="Bool"("DisabledEnum"=w705) -> ()  [unwired: 2 in, 2 out]
            n767 = property on="btn_DSP输入" class="Bool"("DisabledEnum"=w705) -> ()  [unwired: 2 in, 2 out]
            n768 = property on="btn_CAN总线" class="Bool"("DisabledEnum"=w705) -> ()  [unwired: 2 in, 2 out]
            n769 = property on="btn_R232_485总线" class="Bool"("DisabledEnum"=w705) -> ()  [unwired: 2 in, 2 out]
            n770 = property on="btn_LAN总线" class="Bool"("DisabledEnum"=w705) -> ()  [unwired: 2 in, 2 out]
            n771 = property on="btn_自动开始检测类型2" class="Bool"("DisabledEnum"=w705) -> ()  [unwired: 2 in, 2 out]
            n772 = property on="函数类型 1" class="Bool"("DisabledEnum"=w705) -> ()  [unwired: 2 in, 2 out]
            n773 = property on="函数类型 2" class="Bool"("DisabledEnum"=w705) -> ()  [unwired: 2 in, 2 out]
            n774 = property on="函数类型 3" class="Bool"("DisabledEnum"=w705) -> ()  [unwired: 2 in, 2 out]
            n775 = property on="函数类型 4" class="Bool"("DisabledEnum"=w705) -> ()  [unwired: 2 in, 2 out]
          }
        }
      }
    }
    n776 = local read "退出？"() -> (w566:bool)
  }
  n777 = Obtain Notifier(name (unnamed)=w9, notification data type=w9) -> (notifier out=w8:refnum<notifier>, error out=w7:errorcluster)  [unwired: 2 in, 1 out]
  n778 = while {
    tunnel: w8 -> [w720]
    tunnel: w7 -> [w719]
    tunnel: [w718] -> w6
    tunnel: [w717] -> w5
    stop <- w711 stop-if-true
    # "II型板自动测试"
    n779 = Wait Until Next ms Multiple(millisecond multiple=u32 20 ("毫秒倍数")) -> ()  [unwired: 1 out]
    n780 = Wait on Notification(notifier=w720, timeout in ms (-1)=20 ("超时毫秒(-1)"), error in (no error)=w719) -> (notifier out=w718:refnum<notifier>, notification=w715:string, error out=w717:errorcluster)  [unwired: 1 in, 1 out]
    n781 = Equal?(x=w715, y="Auto_2" ("通知")) -> (x = y?=w712:bool)
    n782 = case shown="真" w712 {
      frame False {
      }
      frame True {
        n783 = stacked-sequence {
          frame #0 {
            # "类型1测试"
            n784 = global read "试验配置信息.vi" "测试类型1选择？"() -> (w721:bool)
            n785 = case shown="真" w721 {
              frame False {
              }
              frame True {
                n786 = stacked-sequence {
                  frame #0 {
                    n787 = stacked-sequence {
                      frame #0 {
                        n788 = call "测试类型1自动测试一组.vi"() -> ()  [unwired: 10 in]
                      }
                      frame #1 {
                        n789 = call "自动测试类型1统计结果.vi"() -> ()  [unwired: 12 in]
                      }
                    }
                    n790 = local write "进度提示"("正在进行类型1测试......") -> ()
                  }
                  frame #1 {
                    n791 = global read "试验配置信息.vi" "板卡II自动检测结果"() -> (w726:bool[])
                    n792 = Index Array(array=w726, index=0) -> (element=w724:bool)
                    n793 = case shown="假" w724 {
                      tunnel: [2 1] -> w723
                      frame False {
                      }
                      frame True {
                      }
                    }
                    n794 = case shown="0, 默认" w723 {
                      tunnel: [cluster{u32, u32}[] [{1985280, 1985280}] cluster{u32, u32}[] [{61205, 6618880}] cluster{u32, u32}[] [{16730410, 16711680}]] -> w727
                      frame 0, Default {
                      }
                      frame 1 {
                      }
                      frame 2 {
                      }
                    }
                    n795 = property on="函数类型1检测" class="Bool (严格)"("Colors [4]"=w727) -> ()  [unwired: 2 in, 2 out]
                  }
                }
              }
            }
          }
          frame #1 {
            # "类型2测试"
            n796 = global read "试验配置信息.vi" "测试类型2选择？"() -> (w733:bool)
            n797 = case shown="真" w733 {
              frame False {
              }
              frame True {
                n798 = stacked-sequence {
                  frame #0 {
                    n799 = stacked-sequence {
                      frame #0 {
                        n800 = call "类型2自动测试.vi"() -> ()  [unwired: 12 in]
                      }
                      frame #1 {
                        n801 = call "自动测试类型2统计结果.vi"() -> ()  [unwired: 12 in]
                      }
                    }
                    n802 = local write "进度提示"("正在进行类型2测试......") -> ()
                  }
                  frame #1 {
                    n803 = global read "试验配置信息.vi" "板卡II自动检测结果"() -> (w738:bool[])
                    n804 = Index Array(array=w738, index=1) -> (element=w736:bool)
                    n805 = case shown="假" w736 {
                      tunnel: [2 1] -> w735
                      frame False {
                      }
                      frame True {
                      }
                    }
                    n806 = case shown="0, 默认" w735 {
                      tunnel: [cluster{u32, u32}[] [{1985280, 1985280}] cluster{u32, u32}[] [{61205, 6618880}] cluster{u32, u32}[] [{16730410, 16711680}]] -> w739
                      frame 0, Default {
                      }
                      frame 1 {
                      }
                      frame 2 {
                      }
                    }
                    n807 = property on="函数类型2检测" class="Bool (严格)"("Colors [4]"=w739) -> ()  [unwired: 2 in, 2 out]
                  }
                }
              }
            }
          }
          frame #2 {
            # "类型3测试"
            n808 = global read "试验配置信息.vi" "测试类型3选择？"() -> (w745:bool)
            n809 = case shown="真" w745 {
              tunnel: w745 -> [_ w746]
              frame False {
              }
              frame True {
                n810 = stacked-sequence {
                  tunnel: w746 -> [w748 _]
                  frame #0 {
                    n811 = call "类型3自动测试.vi"("选择?"=w748) -> ()  [unwired: 11 in]
                    n812 = local write "进度提示"("正在进行类型3测试......") -> ()
                  }
                  frame #1 {
                    n813 = global read "试验配置信息.vi" "板卡II自动检测结果"() -> (w752:bool[])
                    n814 = Index Array(array=w752, index=2) -> (element=w750:bool)
                    n815 = case shown="假" w750 {
                      tunnel: [2 1] -> w749
                      frame False {
                      }
                      frame True {
                      }
                    }
                    n816 = case shown="0, 默认" w749 {
                      tunnel: [cluster{u32, u32}[] [{1985280, 1985280}] cluster{u32, u32}[] [{61205, 6618880}] cluster{u32, u32}[] [{16730410, 16711680}]] -> w753
                      frame 0, Default {
                      }
                      frame 1 {
                      }
                      frame 2 {
                      }
                    }
                    n817 = property on="函数类型3检测" class="Bool (严格)"("Colors [4]"=w753) -> ()  [unwired: 2 in, 2 out]
                  }
                }
              }
            }
          }
          frame #3 {
            # "类型4测试"
            n818 = global read "试验配置信息.vi" "测试类型4选择？"() -> (w759:bool)
            n819 = case shown="真" w759 {
              frame False {
              }
              frame True {
                n820 = stacked-sequence {
                  frame #0 {
                    n821 = local write "进度提示"("正在进行类型4测试......") -> ()
                  }
                  frame #1 {
                    n822 = global read "试验配置信息.vi" "板卡II自动检测结果"() -> (w764:bool[])
                    n823 = Index Array(array=w764, index=3) -> (element=w762:bool)
                    n824 = case shown="假" w762 {
                      tunnel: [2 1] -> w761
                      frame False {
                      }
                      frame True {
                      }
                    }
                    n825 = case shown="0, 默认" w761 {
                      tunnel: [cluster{u32, u32}[] [{1985280, 1985280}] cluster{u32, u32}[] [{61205, 6618880}] cluster{u32, u32}[] [{16730410, 16711680}]] -> w765
                      frame 0, Default {
                      }
                      frame 1 {
                      }
                      frame 2 {
                      }
                    }
                    n826 = property on="函数类型4检测" class="Bool (严格)"("Colors [4]"=w765) -> ()  [unwired: 2 in, 2 out]
                  }
                }
              }
            }
          }
          frame #4 {
            # "统计合格率"
            n827 = call "二型板自动测试合格率统计.vi"() -> ()  [unwired: 12 in]
          }
          frame #5 {
            # "报告存储"
            n828 = flat-sequence {
              tunnel: [w772] -> w771
              tunnel: w771 -> [w775]
              frame #0 {
                n829 = Get Date/Time In Seconds() -> (seconds since 1Jan1904=w772:timestamp)
                n830 = call "二型板测试报告存储.vi"("生成报告?"=FALSE, "是否存储到数据库?"=TRUE, "试验时间"=w772) -> ()  [unwired: 9 in]
              }
              frame #1 {
                n831 = global read "自动测试结果.vi" "自测总概述 temp"() -> (w777:string)
                n832 = call "完成2"("Message"=w777) -> ("生成报告"=w776:bool)  [unwired: 9 in, 1 out]
                n833 = case shown="真" w776 {
                  tunnel: w775 -> [_ w778]
                  frame False {
                  }
                  frame True {
                    n834 = call "二型板测试报告存储.vi"("生成报告?"=TRUE, "是否存储到数据库?"=FALSE, "试验时间"=w778) -> ()  [unwired: 9 in]
                  }
                }
              }
            }
          }
          frame #6 {
            w782 = T3."Enabled" ("禁用")
            n835 = case shown="0, 默认" 0 {
              tunnel: [cluster{u32, u32}[] [{1985280, 1985280}] cluster{u32, u32}[] [{61205, 6618880}] cluster{u32, u32}[] [{16730410, 16711680}]] -> w784
              frame 0, Default {
              }
              frame 1 {
              }
              frame 2 {
              }
            }
            n836 = property on="函数类型1检测" class="Bool (严格)"("Colors [4]"=w784) -> ()  [unwired: 2 in, 2 out]
            n837 = property on="函数类型2检测" class="Bool (严格)"("Colors [4]"=w784) -> ()  [unwired: 2 in, 2 out]
            n838 = property on="函数类型3检测" class="Bool (严格)"("Colors [4]"=w784) -> ()  [unwired: 2 in, 2 out]
            n839 = property on="函数类型4检测" class="Bool (严格)"("Colors [4]"=w784) -> ()  [unwired: 2 in, 2 out]
            n840 = local write "进度提示"("测试完毕......") -> ()
            n841 = property on="btn_数字输入" class="Bool"("DisabledEnum"=w782) -> ()  [unwired: 2 in, 2 out]
            n842 = property on="btn_数字输出" class="Bool"("DisabledEnum"=w782) -> ()  [unwired: 2 in, 2 out]
            n843 = property on="btn_DSP输入" class="Bool"("DisabledEnum"=w782) -> ()  [unwired: 2 in, 2 out]
            n844 = property on="btn_CAN总线" class="Bool"("DisabledEnum"=w782) -> ()  [unwired: 2 in, 2 out]
            n845 = property on="btn_R232_485总线" class="Bool"("DisabledEnum"=w782) -> ()  [unwired: 2 in, 2 out]
            n846 = property on="btn_LAN总线" class="Bool"("DisabledEnum"=w782) -> ()  [unwired: 2 in, 2 out]
            n847 = property on="函数类型 1" class="Bool"("DisabledEnum"=w782) -> ()  [unwired: 2 in, 2 out]
            n848 = property on="函数类型 2" class="Bool"("DisabledEnum"=w782) -> ()  [unwired: 2 in, 2 out]
            n849 = property on="函数类型 3" class="Bool"("DisabledEnum"=w782) -> ()  [unwired: 2 in, 2 out]
            n850 = property on="函数类型 4" class="Bool"("DisabledEnum"=w782) -> ()  [unwired: 2 in, 2 out]
            n851 = property on="btn_开始检测" class="Bool"("DisabledEnum"=w782) -> ()  [unwired: 2 in, 2 out]
          }
        }
      }
    }
    n852 = local read "退出？"() -> (w711:bool)
  }
  n853 = Release Notifier(notifier=w11, error in (no error)=w10) -> ()  [unwired: 1 in, 3 out]
  n854 = Release Notifier(notifier=w6, error in (no error)=w5) -> ()  [unwired: 1 in, 3 out]
